vi "Master.vi"() -> ()   [LabVIEW 2025]
doc: "Author: Scott Hannahs <sth@magnet.fsu.edu>\n\nThis software is licensed for use under the “MIT License\"\nCopyright (c) 2025 Scott Hannahs, sth@sth@magnet.sthnet.net\n\nPermission is hereby granted, free of charge, to any person obtaining a copy of this software and associated documentation files (the \"Software\"), to deal in the Software without restriction, including without limitation the rights to use, copy, modify, merge, publish, distribute, sublicense, and/or sell copies of the Software, and to permit persons to whom the Software is furnished to do so, subject to the following conditions: The above copyright notice and this permission notice shall be included in all copies or substantial portions of the Software.\n\nTHE SOFTWARE IS PROVIDED \"AS IS\", WITHOUT WARRANTY OF ANY KIND, EXPRESS OR IMPLIED, INCLUDING BUT NOT LIMITED TO THE WARRANTIES OF MERCHANTABILITY, FITNESS FOR A PARTICULAR PURPOSE AND NONINFRINGEMENT. IN NO EVENT SHALL THE AUTHORS OR COPYRIGHT HOLDERS BE LIABLE FOR ANY CLAIM, DAMAGES OR OTHER LIABILITY, WHETHER IN AN ACTION OF CONTRACT, TORT OR OTHERWISE, ARISING FROM, OUT OF OR IN CONNECTION WITH THE SOFTWARE OR THE USE OR OTHER DEALINGS IN THE SOFTWARE."
uses:
  Globals and TypeDefs/Type Definitions.llb/CCDParameter.ctt
  Globals and TypeDefs/Type Definitions.llb/FileFormatParameter.ctt
  Globals and TypeDefs/Type Definitions.llb/FilePathParameter.ctt
  Globals and TypeDefs/Type Definitions.llb/FileInfoParameter.ctt
  Globals and TypeDefs/Type Definitions.llb/Wavelength Unit.ctt
  Globals and TypeDefs/Type Definitions.llb/McPherson Grating Density.ctl
  Globals and TypeDefs/Type Definitions.llb/OperationMode.ctt
  Globals and TypeDefs/Type Definitions.llb/ListOfDetectors.ctt
  Globals and TypeDefs/Type Definitions.llb/3 way Status.ctl
  LV7/OpticsSS.ctl
  LV7/PlottSS.ctl
  Globals and TypeDefs/gStatus.vi
  Instance          41 14Saved   Master .vi
  Globals and TypeDefs/gDetector.vi
  Globals and TypeDefs/gGeneral.vi
  Sub VIs/File and save/X-Axis Converter.llb/X-Axis Converter.vi
  Globals and TypeDefs/gHField.vi
panel:
  in  "Case Constant\n(See Context Help) 2":bool=TRUE
  in  "Case Constant\n(See Context Help)":bool
  in  "Stop-All":bool
  in  "Prefix_indexed":bool
  out "Path array":path[](array[path])
  out "PDA Temperature":dbl(graph)
  out "#PixelOverflow":u32
  out "Pixel Overflow":bool
  out "Error":errorcluster
  out "Master State":T1=enum."Init"
  in  "EngageTime":bool
  in  "ExpTimeTarget":dbl=12.0
  in  "SaveData?":bool
  in  "Print?":bool
  out "Operation Mode":T2
  in  "SubFolderNamesArray":string[](array[string])
  in  "HTL Array":dbl[][](array[numeric])
  in  "LoadData?":bool
  out "Field":T3 caption="H" items=["N.A.", "OK", "Busy", "Done"]
  out "Tmeperature":T3 caption="T" items=["N.A.", "OK", "Busy", "Done"]
  out "Spectrometer":T3 caption="l" items=["N.A.", "OK", "Busy", "Done"]
  out "Exposure time display":dbl(slide)=0.133 caption="Exposure" scale=0.0..0.2 scale format="%.1f"
  out "Elapsed Time":string
  out "Status Message Board":string="Welcome to NHMFL!\nVisible Optics\nProgram"
  in  "Check Prefix?":bool
  in  "SetDirectory?":bool
  in  "Y Data":dbl[](array[numeric])=[4.359859227115864, 4.389200892828675, 4.418863708420512, 4.448852482615925, 4.479172114380057, 4.509827594937488, 4.540824009842933, 4.572166541105726, 4.6038604693694944, 4.635911176148454, 4.668324146122441, 4.701104969491852, 4.734259344394734, 4.767793079387671, 4.801712095992179, 4.83602243130902, 4.870730240701915, 4.905841800553186, 4.941363511093324, 4.97730189930649, 5.0136636219147634, 5.050455468442887, 5.087684364366512, 5.125357374346244, 5.16348170554992, 5.202064711066347, 5.241113893412698, 5.280636908138933, 5.320641567532123, 5.361135844423454, 5.40212787610175, 5.443625968336108, 5.485638599511655, 5.528174424881744, 5.571242280940019, 5.614851189916724, 5.659010364402478, 5.703729212104152, 5.749017340736845, 5.79488456305601, 5.8413409020348865, 5.888396596191121, 5.936062105068024, 5.984348114875219, 6.033265544293544, 6.082825550450229, 6.133039535069095, 6.1839191508021365, 6.235476307748183, 6.287723180164464, 6.340672213378188, 6.394336130903802, 6.44872794177352, 6.5038609480878895, 6.55974875279337, 6.616405267695311, 6.673844721713221, 6.732081669387259, 6.79113099964405, 6.851007944830221, 6.9117280900235425, 6.9733073826300265, 7.0357621422775445, 7.099109071015688, 7.1633652638319365, 7.228548219495836, 7.294675851741292, 7.36176650079951, 7.429838945294219, 7.498912414511272, 7.569006601056504, 7.640141673914049, 7.7123382919199805, 7.785617617665268, 7.860001331842512, 7.935511648052952, 8.012171328088485, 8.090003697706326, 8.169032662913095, 8.249282726775652, 8.33077900677827, 8.413547252743905, 8.49761386534048, 8.58300591519227, 8.66975116261715, 8.757878078012872, 8.847415862913794, 8.93839447174277, 9.030844634282277, 9.124797878889435, 9.220286556482478, 9.317343865324164, 9.41600387663149, 9.516301561040184, 9.618272815953393, 9.721954493806981, 9.827384431281825, 9.934601479497585, 10.043645535221685, 10.154557573128157, 10.267379679144385, 10.382155084921548, 10.498928203469083, 10.617744665992642, 10.738651359976075, 10.861696468551548, 10.986929511199559, 11.114401385825383, 11.244164412257609, 11.376272377215363, 11.510780580794803, 11.647745884522498, 11.787226761028752, 11.929283345392315, 12.073977488209161, 12.22137281044176, 12.371534760102007, 12.524530670826199, 12.680429822398747, 12.83930350328164, 13.001225075210728, 13.166270039915263, 13.33451610802253, 13.506043270206384, 13.680933870638214, 13.859272682802093, 14.041146987729777, 14.226646654715656, 14.41586422456719, 14.608894995444231, 14.80583711134241, 15.00679165326711, 15.211862733147012, 15.421157590528683, 15.634786692088575, 15.852863833997525, 16.075506247159804, 16.302834705347756, 16.534973636240313, 16.77205123536335, 17.014199582923293, 17.261554763504943, 17.51425698859712, 17.77245072188844, 18.036284807256397, 18.3059125993568, 18.58149209668873, 18.863186076991337, 19.15116223479378, 19.445593320905605, 19.746657283603096, 20.054537411216362, 20.369422475784297, 20.691506877387, 21.02099078870748, 21.35808029931693, 21.702987559097092, 22.0559309201451, 22.417135076413132, 22.786831200239348, 23.165257074828247, 23.552657221611106, 23.949283021300772, 24.35539282730692, 24.771252070023422, 25.197133350337953, 25.63331652051566, 26.080088750418582, 26.537744576792313, 27.006585933108887, 27.486922157200187, 27.979069973614642, 28.48335344733274, 29.000103905129734, 29.52965982050742, 30.072366657732513, 30.628576670076946, 31.198648646914766, 31.78294760382926, 32.38184440935961, 32.99571534146977, 33.624941566211746, 34.26990853044752, 34.931005259824005, 35.60862355250491, 36.3031570584605, 37.01500023335454, 37.74454715533088, 38.49219019221989, 39.25831850591429, 40.04331637991872, 40.847561355318334, 41.67142215974196, 42.51525641324812, 43.37940809451772, 44.26420475032537, 45.169954430957425, 46.09694233418251, 47.04542714051036, 48.015637022906574, 49.00776531492666, 50.02196582239054, 51.05834776541544, 52.11697033983435, 53.19783688989854, 54.30088868779076, 55.42599831987955, 56.57296268504168, 57.74149561674433, 58.931220148080584, 60.1416604476788, 61.37223346434939, 62.622240329675115, 63.890857580390986, 65.17712827640742, 66.4799531056599, 67.79808158341963, 69.1301034712415, 70.47444055896403, 71.82933897185566, 73.19286218368788, 74.56288493456158, 75.93708826921247, 77.31295592634606, 78.68777232151824, 80.05862237420615, 81.42239343285824, 82.77577954893358, 84.11528834098996, 85.43725067181454, 86.73783333448564, 88.0130549062849, 89.25880488223545, 90.4708661424704, 91.64494074005955, 92.77667891917588, 93.86171118887495, 94.89568318741601, 95.87429297840674, 96.79333032630886, 97.64871740856572, 98.43655033863818, 99.15314080272404, 99.79505705677101, 100.35916349333694, 100.84265797303367, 101.24310612502882, 101.55847185679316, 101.78714337508754, 101.92795410705088, 101.98019801980197, 101.94363896561752, 101.81851382289437, 101.60552935527126, 101.30585286653462, 100.92109688110092, 100.4532982230126, 99.90489199503531, 99.27868106899476, 98.57780178535918, 97.80568662187997, 96.96602462681605, 96.06272042200558, 95.09985256623146, 94.08163203227065, 93.01236149485176, 91.89639605523514, 90.73810594515385, 89.54184166257876, 88.31190189802533, 87.05250451647399, 85.76776076963034, 84.461652828644, 83.13801465065819, 81.8005161249856, 80.4526503871352, 79.09772414177037, 77.73885079871027, 76.37894619898024, 75.02072668985214, 73.66670929786417, 72.31921374603169, 70.98036606460397, 69.65210355285129, 68.33618086133153, 67.03417697891065, 65.74750292571056, 64.47740997120414, 63.22499821536264, 61.99122538944135, 60.77691575122682, 59.582768967111335, 58.40936888981143, 57.25719215587677, 56.12661654114332, 55.017929024924804, 53.93133352507879, 52.86695827602707, 51.82486283053664, 50.80504467356964, 49.807445442875476, 48.831956756394504, 47.87842565094678, 46.94665964030745, 46.036431403641515, 45.14748311748012, 44.27953044611727, 43.43226620646358, 42.6053637241895, 41.79847989842212, 41.011257992390064, 40.243330167348105, 39.49431977680977, 38.763843437704175, 38.05151289452863, 37.356936691921696, 36.67972167041139, 36.01947429933415, 35.37580186017517, 34.74831349280977, 34.13662111634363, 33.540340235512275, 32.959090642839186, 32.39249702604861, 31.840189489538492, 31.301803998049735, 30.7769827500592, 30.265374487814174, 29.76663475037882, 29.28042607553899, 28.80641815591104, 28.344287954158954, 27.893719781782664, 27.454405345555568, 27.026043765322786, 26.608341566525006, 26.201012650514798, 25.803778245431467, 25.41636684014538, 25.03851410354023, 24.669962791171823, 24.31046264115136, 23.95977026090333, 23.61764900628636, 23.28386885441087, 22.95820627133951, 22.640444075739502, 22.330371299429107, 22.027783045661604, 21.73248034589445, 21.444270015698585, 21.16296451039404, 20.888381780917932, 20.620345130372943, 20.35868307164673, 20.10322918643533, 19.853821985965663, 19.61030477366188, 19.372525509968213, 19.140336679507016, 18.913595160715975, 18.692162098089153, 18.475902777115053, 18.26468650198858, 18.058386476154528, 17.856879685719345, 17.660046785759945, 17.467771989538537, 17.279942960625498, 17.09645070792191, 16.917189483561163, 16.742056683667286, 16.570952751935298, 16.403781085997196, 16.240447946532107, 16.080862369071976, 15.924936078455998, 15.772583405879114, 15.623721208481035, 15.478268791420303, 15.336147832373733, 15.197282308405232, 15.061598425142755, 14.929024548204785, 14.799491136817574, 14.672930679561734, 14.549277632191464, 14.428468357465825, 14.310441066935024, 14.195135764625045, 14.08249419256267, 13.972459778087526, 13.864977582895126, 13.759994253758327, 13.657457974875705, 13.557318421794335, 13.459526716859063, 13.364035386138228, 13.27079831777925, 13.179770721748449, 13.090909090909092, 13.004171163395661, 12.91951588624077, 12.836903380214224, 12.75629490583483, 12.677652830515154, 12.600940596803213, 12.526122691683634, 12.453164616903683, 12.38203286029049, 12.312694868025606, 12.24511901784625, 12.179274593141457, 12.115131757913815, 12.05266153257834, 11.99183577056985, 11.932627135733041, 11.87500908046845, 11.818955824609674, 11.76444233500797, 11.711444305800104, 11.65993813933795, 11.60990092775727, 11.561310435165108, 11.514145080425847, 11.468383920525726, 11.424006634497912, 11.380993507889265, 11.339325417751663, 11.298983818141277, 11.259950726108972, 11.222208708166901, 11.185740867215678, 11.150530829917827, 11.116562734503766, 11.083821218996304, 11.052291409841342, 11.021958910931758, 10.992809793012693, 10.964830583456795, 10.938008256397914, 10.912330223212965, 10.887784323341283, 10.864358815431716, 10.842042368808027, 10.820824055243078, 10.800693341033405, 10.781640079365355, 10.763654502964759, 10.746727217022421, 10.730849192387653, 10.716011759022894, 10.702206599712252, 10.689425744017434, 10.677661562474725, 10.666906761026693, 10.657154375683012, 10.648397767404552, 10.640630617205472, 10.633846921468175, 10.628040987466086, 10.623207429089685, 10.619341162771164, 10.616437403603506, 10.61449166164985, 10.613499738439238, 10.613457723645045, 10.614361991942566, 10.616209200042398, 10.61899628389644, 10.622720456073516, 10.627379203301786, 10.632970284175236, 10.639491727021781, 10.646941827930538, 10.65531914893617, 10.664622516358094, 10.674851019292753, 10.68600400825716, 10.698081093981964, 10.711082146352725, 10.725007293497864, 10.73985692102218, 10.755631671384794, 10.77233244342051, 10.789960392003877, 10.808516927855083, 10.828003717487244, 10.848422683294594, 10.869776003781105, 10.892066113929618, 10.91529570571105, 10.939467728734005, 10.96458539103486, 10.990652160008423, 11.01767176347996, 11.045648190918651, 11.074585694793534, 11.104488792072516, 11.135362265865236, 11.167211167211168, 11.20004081701363, 11.233856808121402, 11.268665007559191, 11.304471558908258, 11.341282884839375, 11.379105689799312, 11.41794696285327, 11.457813980685149, 11.498714310757618, 11.540655814634878, 11.583646651469962, 11.62769528165972, 11.672810470670129, 11.719001293034513, 11.766277136528466, 11.814647706523917, 11.864123030526423, 11.914713462898968, 11.966429689775758, 12.019282734170648, 12.073283961283387, 12.12844508400873, 12.184778168652574, 12.242295640859474, 12.301010291757152, 12.360935284322133, 12.42208415997257, 12.48447084539341, 12.548109659599271, 12.613015321241827, 12.679202956166797, 12.746688105227863, 12.815486732363786, 12.885615232945288, 12.957090442399794, 13.029929645120367, 13.104150583667508, 13.179771468271484, 13.256810986643078, 13.335288314102453, 13.415223124033782, 13.496635598676047, 13.579546440259186, 13.66397688249509, 13.749948702434974, 13.837484232702424, 13.926606374114439, 14.017338608701486, 14.109705013137976, 14.203730272596845, 14.299439695039455, 14.396859225955392, 14.4960154635654, 14.596935674501095, 14.699647809977643, 14.804180522472912, 14.910563182930376, 15.018825898501593, 15.128999530844538, 15.241115714996932, 15.355206878840859, 15.471306263179047, 15.589447942441705, 15.709666846043369, 15.831998780412336, 15.956480451712276, 16.08314948928004, 16.212044469802226, 16.343204942253628, 16.47667145362424, 16.612485575458262, 16.750689931233456, 16.89132822460762, 17.034445268559747, 17.180087015457268, 17.328300588077308, 17.479134311615432, 17.632637746713556, 17.78886172353971, 17.9478583769566, 18.109681182812103, 18.274384995391078, 18.442026086065923, 18.612662183184362, 18.786352513237837, 18.963157843349737, 19.143140525129375, 19.326364539935806, 19.51289554559672, 19.70280092463277, 19.896149834033558, 20.09301325663871, 20.29346405417522, 20.49757702200397, 20.705428945633606, 20.917098659055448, 21.13266710496104, 21.35221739690145, 21.57583488344913, 21.803607214428858, 22.03562440927946, 22.27197892761611, 22.51276574206055, 22.758082413407966, 23.008029168205347, 23.262708978810554, 23.522227646009927, 23.786693884269244, 24.056219409693583, 24.3309190307785, 24.610910742027375, 24.896315820519412, 25.187258925508026, 25.483868201129862, 25.786275382310958, 26.09461590394749, 26.409029013447665, 26.729657886715053, 27.05664974765271, 27.39015599127249, 27.73033231048255, 28.077338826633632, 28.431340223896083, 28.79250588753546, 29.161010046158022, 29.537031917981217, 29.920755861189793, 30.31237152842447, 30.71207402544193, 31.120064073983663, 31.536548178868856, 31.961738799326668, 32.395854524562374, 32.83912025353589, 33.291767378922756, 33.75403397519474, 34.22616499074848, 34.70841244397801, 35.20103562315853, 35.70430128998762, 36.21848388658109, 36.743865745697, 37.2807373039094, 37.82939731740552, 38.39015308003834, 38.96332064319138, 39.54922503696516, 40.14820049211286, 40.76059066207344, 41.386748844375965, 42.0270382005743, 42.681831973785435, 43.35151370277646, 44.03647743141852, 44.73712791219888, 45.453880802309456, 46.18716285068311, 46.937412074152704, 47.705077920707076, 48.49062141761412, 49.29451530191956, 50.11724413059322, 50.95930436729756, 51.821204442444625, 52.70346478289072, 53.60661780723075, 54.53120788228832, 55.47779123595873, 56.44693582110416, 57.43922112472759, 58.45523791609419, 59.495587926931485, 60.56088345621398, 61.651746891388925, 62.76881013723119, 63.91271394274945, 65.08410711582407, 66.28364561441893, 67.51199150234996, 68.76981175672066, 70.05777691316518, 71.37655953411455, 72.72683248428955, 74.1092669966185, 75.52453051079203, 76.97328426561938, 78.45618062540582, 79.97386011959668, 81.52694817404465, 83.11605151148629, 84.7417541980828, 86.4046133123965, 88.10515421280739, 89.84386537927608, 91.62119280559367, 93.43753391876069, 95.29323100317171, 97.1885641087292, 99.12374342407416, 101.0989010989011, 103.11408250278154, 105.16923691237619, 107.26420762426427, 109.39872149710654, 111.5723779346085, 113.78463732972462, 116.03480900108816, 118.32203866462099, 120.64529549690151, 123.0033588622068, 125.39480479205825, 127.81799232482636, 130.27104983316252, 132.75186148874656, 135.25805403686783, 137.78698407721993, 140.33572607186628, 142.90106132583995, 145.47946820982128, 148.0671139170434, 150.65984806694533, 153.2531984854103, 155.84236950429036, 158.4222431302903, 160.98738343390016, 163.53204450143193, 166.05018227635358, 168.53547058854588, 170.9813216309795, 173.38091109184288, 175.72720808570307, 178.01300995009646, 180.23098188419874, 182.37370130512846, 184.43370668665264, 186.40355052675318, 188.27585596792636, 190.0433764705767, 191.6990578197283, 193.23610163304818, 194.64802943849332, 195.92874630773915, 197.0726029712699, 198.0744553067754, 198.92972008756837, 199.6344259043045, 200.1852582325435, 200.5795977101961, 200.81555081101075, 200.89197224975223, 200.80847862709987, 200.5654530119324, 200.16404035900476, 199.60613386401218, 198.89435255837313, 198.0320106357045, 197.02307917433632, 195.87214106971265, 194.58434011263304, 193.16532524079693, 191.6211910503684, 189.95841568084745, 188.18379718160273, 186.30438943418605, 184.32743864427007, 182.2603213348983, 180.11048467305204, 177.885389849312, 175.5924591102524, 173.23902691969622, 170.83229560237197, 168.37929570520407, 165.88685120068226, 163.3615495556608, 160.8097165991903, 158.23739604580024, 155.6503334662017, 153.0539644459122, 150.45340663317825, 147.85345535000155, 145.25858242321343, 142.67293788490863, 140.10035419216482, 137.5443526233475, 135.0081515211617, 132.4946760699316, 130.0065693149577, 127.54620415450763, 125.11569605897792, 122.71691629626862, 120.35150546699153, 118.0208871769936, 115.72628169770708, 113.46871948655841, 111.24905445988026, 109.06797692949733, 106.92602613107003, 104.82360228761749, 102.76097816526601, 100.7383100902379, 98.7556484066402, 96.81294736358653, 94.91007442793571, 93.04681902541851, 91.22290071827247, 89.43797683196064, 87.69164954700636, 85.98347247475698, 84.31295673795266, 82.67957657842356, 81.08277451527354, 79.52196607740966, 77.99654413451097, 76.50588285043271, 75.04934128267388, 73.62626665105351, 72.23599729800955, 70.87786536216365, 69.55119918590644, 68.25532547678353, 66.989571241518, 65.75326551045683, 64.54574086924336, 63.36633481351214, 62.21439094139057, 61.089259997666595, 59.99030078251254, 58.91688093678181, 57.8683776150366, 56.84417805662603, 55.84368006439242, 54.86629239981791, 53.911435102754524, 52.97853974323218, 52.06704961221306, 51.17641985762386, 50.306117571439195, 49.45562183311679, 48.624423714227504, 47.812026248683935, 47.01794437260552, 46.24170483747118, 45.48284609989282, 44.74091819103539, 44.01548256841131, 43.306111952540896, 42.61239015070839, 41.933911869839505, 41.270282520325516, 40.62111801242236, 39.986044546706715, 39.364698399897456, 38.75672570722455, 38.16178224240005, 37.579533196118035, 37.0096529539243, 36.451824874181916, 35.90574106678451, 35.37110217318958, 34.847617148262465, 34.335003044374055, 33.83298479812016, 33.341295019989, 32.85967378725514, 32.38786844032609, 31.92563338274469, 31.472729885000874, 31.028925892285255, 30.59399583628902, 30.167720451121262, 29.749886593406902, 29.340287066594833, 28.938720449497826, 28.54499092906973, 28.15890813740441, 27.780286992941413, 27.408947545840558, 27.044714827486775, 26.687418704078205, 26.3368937342368, 25.992979030586355, 25.65551812522657, 25.324358839035185, 24.999353154726343, 24.680357093584345, 24.367230595799825, 24.059837404323954, 23.758044952161082, 23.461724253019675, 23.170749795234723, 22.884999438884304, 22.60435431601352, 22.328698733885684, 22.05792008118085, 21.791908737057103, 21.53055798299983, 21.27376391737627, 21.021425372619895, 20.773443834969687, 20.529723366686287, 20.290170530675923, 20.054694317446987, 19.82320607433054, 19.595619436897397, 19.371850262501688, 19.151816565889344, 18.93543845680471, 18.722638079534455, 18.513339554329608, 18.30746892064386, 18.104954082134622, 17.90572475336819, 17.709712408176312, 17.51685022961275, 17.327073061456208, 17.140317361213445, 16.956521154571956, 16.77562399125692, 16.597566902248243, 16.42229235831149, 16.249744229803607, 16.07986774770962, 15.912609465871899, 15.747917224374362, 15.585740114042, 15.4260284420226, 15.26873369841338, 15.113808523899822, 14.961206678374843, 14.810883010504563, 14.662793428212746, 14.51689487005212, 14.373145277435007, 14.231503567696258, 14.091929607959841, 13.954384189785666, 13.818829004569535, 13.685226619673003, 13.553540455260446, 13.423734761818881, 13.295774598341003, 13.169625811148363, 13.045255013335167, 12.922629564813562, 12.801717552939623, 12.682487773703725, 12.56490971346569, 12.448953531218253, 12.334590041362802, 12.221790696979657, 12.110527573579299, 12.000773353317886, 11.892501309663155, 11.785685292497277, 11.68029971364149, 11.5763195327913, 11.4737202438479, 11.372477861634222, 11.272568908984288, 11.173970404192929, 11.076659848816483, 10.980615215812294, 10.885814938007247, 10.792237896885748, 10.699863411686152, 10.608671228797805, 10.518641511448305, 10.429754829672692, 10.341992150556594, 10.255334828743806, 10.169764597201846, 10.085263558236575, 10.001814174748855, 9.919399261726573, 9.838001977963811, 9.757605818001839, 9.678194604284215, 9.599752479520156, 9.522263899250422, 9.445713624608777, 9.370086715274489, 9.295368522609328, 9.22154468297399, 9.148601111219307, 9.076523994345967, 9.00529978532927, 8.934915197103027, 8.865357196698499, 8.79661299953429, 8.728670063851933, 8.661516085294144, 8.595138991620736, 8.529526937558694, 8.464668299782959, 8.400551672023308, 8.337165860294927, 8.274499878248228, 8.212542942635004, 8.151284468887964, 8.090714066809685, 8.030821536368922, 7.971596863600483, 7.913030216606138, 7.855111941654126, 7.797832559373704, 7.741182761043143, 7.685153404967791, 7.629735512946082, 7.574920266821415, 7.520699005116799, 7.467063219750945, 7.4140045528328695, 7.361514793533171, 7.309585875030267, 7.258209871528803, 7.207378995349226, 7.157085594085887, 7.107322147832155, 7.058081266471045, 7.009355687028948, 6.961138271091613, 6.913422002280089, 6.866199983785316] format="%.4f"
  in  "File Info":T4={"FilePath"=path "/Volumes/DATA/Labview Items", "Field (T)"=55.0, "Temperature (K)"=77.0, "X-Axis"=enum."nm", "Center nm"=55.0, "Current Grating Density"=enum."600", "CCD Parameters"={"Exposure Time (s)"=0.2, "Offset"=0.0, "BkgrdCrct"=FALSE, "Shutter"=FALSE, "Mode"=enum."Regular", "Repetition"=4, "dt or s"=0.0}, "Operation Mode"=enum."NML Data Acquisition", "Exp Index"=0, "Index_repetition"=0, "Index"=0, "Current Detector"=enum."CCD-1024x256"} {"CCD Parameters"."dt or s" format="%#.6f"; "CCD Parameters"."Repetition" min=1; "CCD Parameters"."Offset" format="%#.2f"; "CCD Parameters"."Exposure Time (s)" min=0.02 max=6000.0 format="%#.2f"; "Center nm" format="%.2f"; "Temperature (K)" format="%.2f"; "Field (T)" format="%.2f"}
  out "Most recently saved file":path=path "erererere"
  in  "FilePath_C":T9={"Filename Prefix"="MyData", "Extension"=enum."±Field", "Suffix"="", "Current Path"=path "/Volumes/Cell06DataMac/Users/Shared/Data"}
  in  "User Comments":string="This data's for you!\nThis is where the experimenter can write random, rambling comments that will never be looked at but will be stored (if you choose so) for all eternity with the data file header."
  in  "Main Tab":T10(tab)
  in  "ShowRange":bool
  in  "CCD Parameters":T7={"Exposure Time (s)"=0.2, "Offset"=580.0, "BkgrdCrct"=FALSE, "Shutter"=TRUE, "Mode"=enum."Regular", "Repetition"=1, "dt or s"=0.0} {"dt or s" format="%#.6f"; "Repetition" min=1; "Offset" format="%#.2f"; "Exposure Time (s)" min=0.02 max=6000.0 format="%#.2f"}
  in  "CCD Control Tab":T11(tab)
  in  "AutoSaveData":bool
  in  "BkgrdShot":bool
  in  "nextShot":bool caption="Shot"
  in  "CancelSeq?":bool
  in  "Park Seq":bool caption="Park after exp?"
  in  "PauseSeq?":bool
  in  "startSeq?":bool
  in  "RampSelect":bool[](array[boolean])=[TRUE, TRUE, FALSE, FALSE, FALSE, FALSE]
  in  "HRamp Paras":dbl[][](array[numeric])=[[0.0, 30.0, 1.0, 20.0], [30.0, 0.0, -1.0, 20.0], [0.0, -30.0, -1.0, 20.0], [-30.0, 0.0, 1.0, 20.0], [0.0, 30.0, 0.5, 20.0], [30.0, 0.0, -0.5, 20.0]] step=1.0 format="%.2f"
  in  "CancelCustSeq?":bool
  in  "Park Cust Seq":bool caption="Park after exp?"
  in  "Cust Seq Para Setup":bool
  in  "PauseCustSeq?":bool
  in  "startCustSeq?":bool
  in  "Init PDA":bool
  in  "Init CCD":bool
  out "InGaAs OK?":bool
  out "CCD OK?":bool
  in  "Select Detector":enum8{"CCD-1024x256", "InGaAs PDA-1024x1"}(ring)
  in  "CCD LineSet?":bool caption="ldb,1,16,u,0,225,25,b,1,15;sdu,0,1024,1024;cl0;omrm;sron"
  in  "Calibration":bool
  in  "Main Setup Tab":enum32{"General Info", "Expert Setup"}(tab)
  in  "File Format":T12={"File Format"=enum."Macintosh (EOL: CR)", "Delimiter"=enum."TAB", "SaveComments?"=enum."Saved in the Header Area"}
  in  "Data Buffer Size":i16=100 min=10 max=500
  in  "BusScan?":bool
  in  "Graph Tab":T13(tab)
  out "File Info Buffer Out":T4[](array[typedef]) {"CCD Parameters"."dt or s" format="%#.6f"; "CCD Parameters"."Repetition" min=1; "CCD Parameters"."Offset" format="%#.2f"; "CCD Parameters"."Exposure Time (s)" min=0.02 max=6000.0 format="%#.2f"; "Center nm" format="%.2f"; "Temperature (K)" format="%.2f"; "Field (T)" format="%.2f"}
  out "Cursor delta x & y":dbl[](array[numeric])
  in  "Fixed":bool
  out "Pin":bool[](array[boolean])=[FALSE, FALSE, FALSE, FALSE, FALSE, FALSE, FALSE, FALSE, FALSE, TRUE]
  in  "Column Headings":string[](array[string])=["Current", "Previous", "older", "Ref#1", "Ref#2", "Ref#3", "Ref#4", "Ref#5", "Ref#6", "Ref#7"]
  in  "Trace":bool[](array[boolean])=[FALSE, FALSE, FALSE, FALSE, FALSE, FALSE, FALSE, FALSE, FALSE, FALSE]
  in  "X-Axis Unit":u16(ring)=1 items=["Point #", "nanometer (nm)", "electron volt (eV)", "Milli eV (meV)", "Wavenumber (cm-1)"]
  out "Main Data Plot":cluster{dbl[], dbl[]}[](graph)
  in  "FindBPeaks":bool
  in  "FindAPeaks":bool
  out "A peaks: X":dbl[](array[numeric]) format="%#_8g"
  out "A peaks: Y":dbl[](array[numeric]) format="%.3e"
  out "B peaks: X":dbl[](array[numeric]) format="%#_8g"
  out "B peaks: Y":dbl[](array[numeric]) format="%.3e"
  in  "APeakIndex":u16(ring)=4 items=[" 1:  693.402 nm", " 2:  694.827 nm"]
  in  "BPeakIndex":u16(ring)=4 items=[" 1:  693.418 nm", " 2:  694.865 nm"]
  out "DX":dbl caption="kb" format="%.2f"
  in  "Pressure Unit?":bool
  out "Analyis Data Plot":cluster{dbl[], dbl[]}[](graph)
  out "Waveform Graph":dbl[](graph)
  out "Op-Mode":u8(ring) items=["none", " + ", " - ", " * ", " / ", "Integral", "Differential", "FFT"]
  in  "Print IntGraph":bool
  in  "Operation":bool
  in  "Ref Load":bool
  in  "Batch Load":bool
  out "Data IntGraph":dbl[][](graph)
  out "Intensity Graph":i32[][](graph)
  # "l"
  # "Filename Prefix"
  # "Extension"
  # "Suffix"
  # "Select   StartField (T)   EndField (T)   FieldStep (T)"
  # "To be constructed"
  # "To be constructed"
  # "Peak#   Position   Intensity"
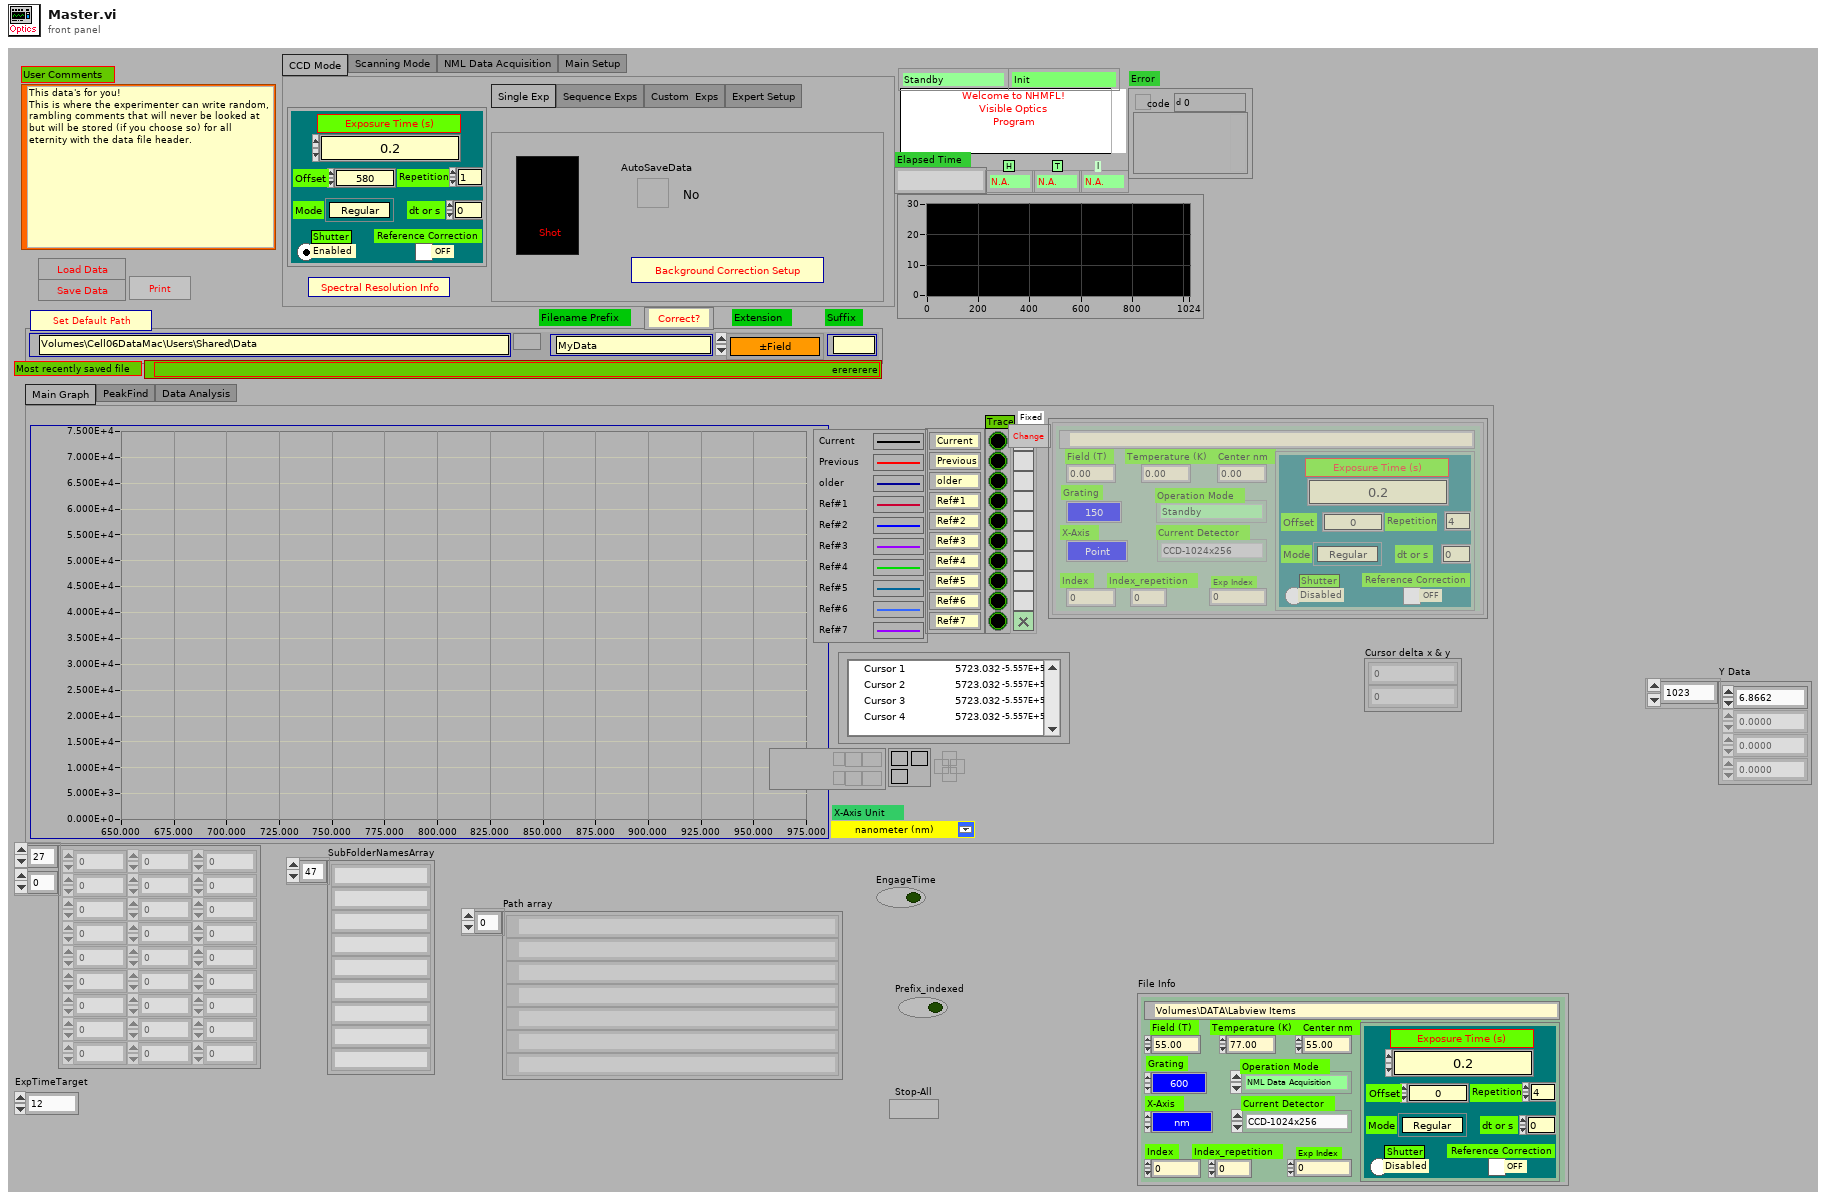
[diagram p1: front panel]
types:
  T1 = typedef "OpticsSS.ctl" = enum16{"_Quit_", "Init", "Ready", "HTL", "CCD_shot", "QueueData", "Error Handler", "HTL Error", "CCD Error", "CCDSetup", "Calibration", "BG_Setup", "HTL Paras Setup"}
  T2 = typedef "OperationMode.ctt" = enum16{"Standby", "CCD Single Shot", "CCD Sequence Shots", "CCD Custom Shots", "CCD Reference Shot", "Step Scanning ", "Time Scanning", "NML Data Acquisition"}
  T3 = typedef "3 way Status.ctl" = u8
  T4 = typedef "FileInfoParameter.ctt" = cluster{"FilePath":path, "Field (T)":dbl, "Temperature (K)":dbl, "X-Axis":T5, "Center nm":dbl, "Current Grating Density":T6, "CCD Parameters":T7, "Operation Mode":T2, "Exp Index":u32, "Index_repetition":u16, "Index":u16, "Current Detector":T8}
  T5 = typedef "Wavelength Unit.ctt" = enum8{"Point", "nm", "eV", "meV", "cm_1"}
  T6 = typedef "McPherson Grating Density.ctl" = enum8{"150", "300", "600", "1200", "1800"}
  T7 = typedef "CCDParameter.ctt" = cluster{"Exposure Time (s)":dbl, "Offset":dbl, "BkgrdCrct":bool, "Shutter":bool, "Mode":enum8{"Regular", "OverExp Cor", "SpikeRemove", "ForCalibration"}, "Repetition":u16, "dt or s":dbl}
  T8 = typedef "ListOfDetectors.ctt" = enum8{"CCD-1024x256", "InGaAs PDA-1024x1", "CCD-1340x400", "Ge Single Channel", "Si Single Channel", "PMT Single Channel"}
  T9 = typedef "FilePathParameter.ctt" = cluster{"Filename Prefix":string, "Extension":enum16{"none", "\".001\",\".002\", ...", "001 (No dot)", "±Field", "pField nField", "Temperature", "Wavelength", "T(K)±H(T)", "(nm)T(K)±H(T)", "User Defined"}, "Suffix":string, "Current Path":path}
  T10 = enum32{"CCD Mode", "Scanning Mode", "NML Data Acquisition", "Main Setup"}
  T11 = enum32{"Single Exp", "Sequence Exps", "Custom  Exps", "Expert Setup"}
  T12 = typedef "FileFormatParameter.ctt" = cluster{"File Format":enum16{"Macintosh (EOL: CR)", "Unix (EOL: LF)", "DOS/Windows (EOL: CR+LF)"}, "Delimiter":enum16{"TAB", "COMMA", "SPACE"}, "SaveComments?":enum16{"Bare data only", "Saved in the Header Area", "Saved as a Parameter File"}}
  T13 = enum32{"Main Graph", "PeakFind", "Data Analysis"}
  T14 = enum16{"--Quit--", "Init GPIB", "Poll GPIB", "Wait for SRQ", "Clear CCD Parameters", "New CCD Parameters", "Check CCD Command Error"}
  T15 = cluster{"Exposure (ms)":u32, "Interval (ms)":u32, "Flush Count":i32, "Trigger":u16}
  T16 = enum16{"End", "Init", "Reset", "SetAcqParameter", "SetArea", "Start Acquisition", "Busy Status Poll", "Read", "Stop"}
  T17 = enum16{"Pass", "Write", "Read", "ReadPlotBlock", "Initialize", "InitFromBufferInput", "Resize Buffer"}
  T18 = enum32{"existing file", "new file", "new or existing file", "existing dir", "new dir", "new or existing dir", "existing file (use LLBs)", "new file (use LLBs)", "new or existing file (use LLBs)", "new or existing file or directory (use LLBs)"}
  T19 = enum16{"none", "\".001\",\".002\", ...", "001 (No dot)", "±Field", "pField nField", "Temperature", "Wavelength", "T(K)±H(T)", "(nm)T(K)±H(T)", "User Defined"}
  T20 = enum16{"none", " + ", " - ", " * ", " / ", "Integral", "Differential", "FFT"}
  T21 = typedef "PlottSS.ctl" = enum16{"_Quit_", "Init", "load", "Pin-Mix", "Trace-Show/Hide", "Unit-Change", "Display/Print", "Column Heading"}
  T22 = enum16{"The Reference CCD Shot", "The Reference File", "The Constant", "Current Reference"}
  T23 = enum16{"Auto Data Saving", "Manual Data Saving", "Auto Sequence Saving", "Sequence Saving from Data Buffer"}
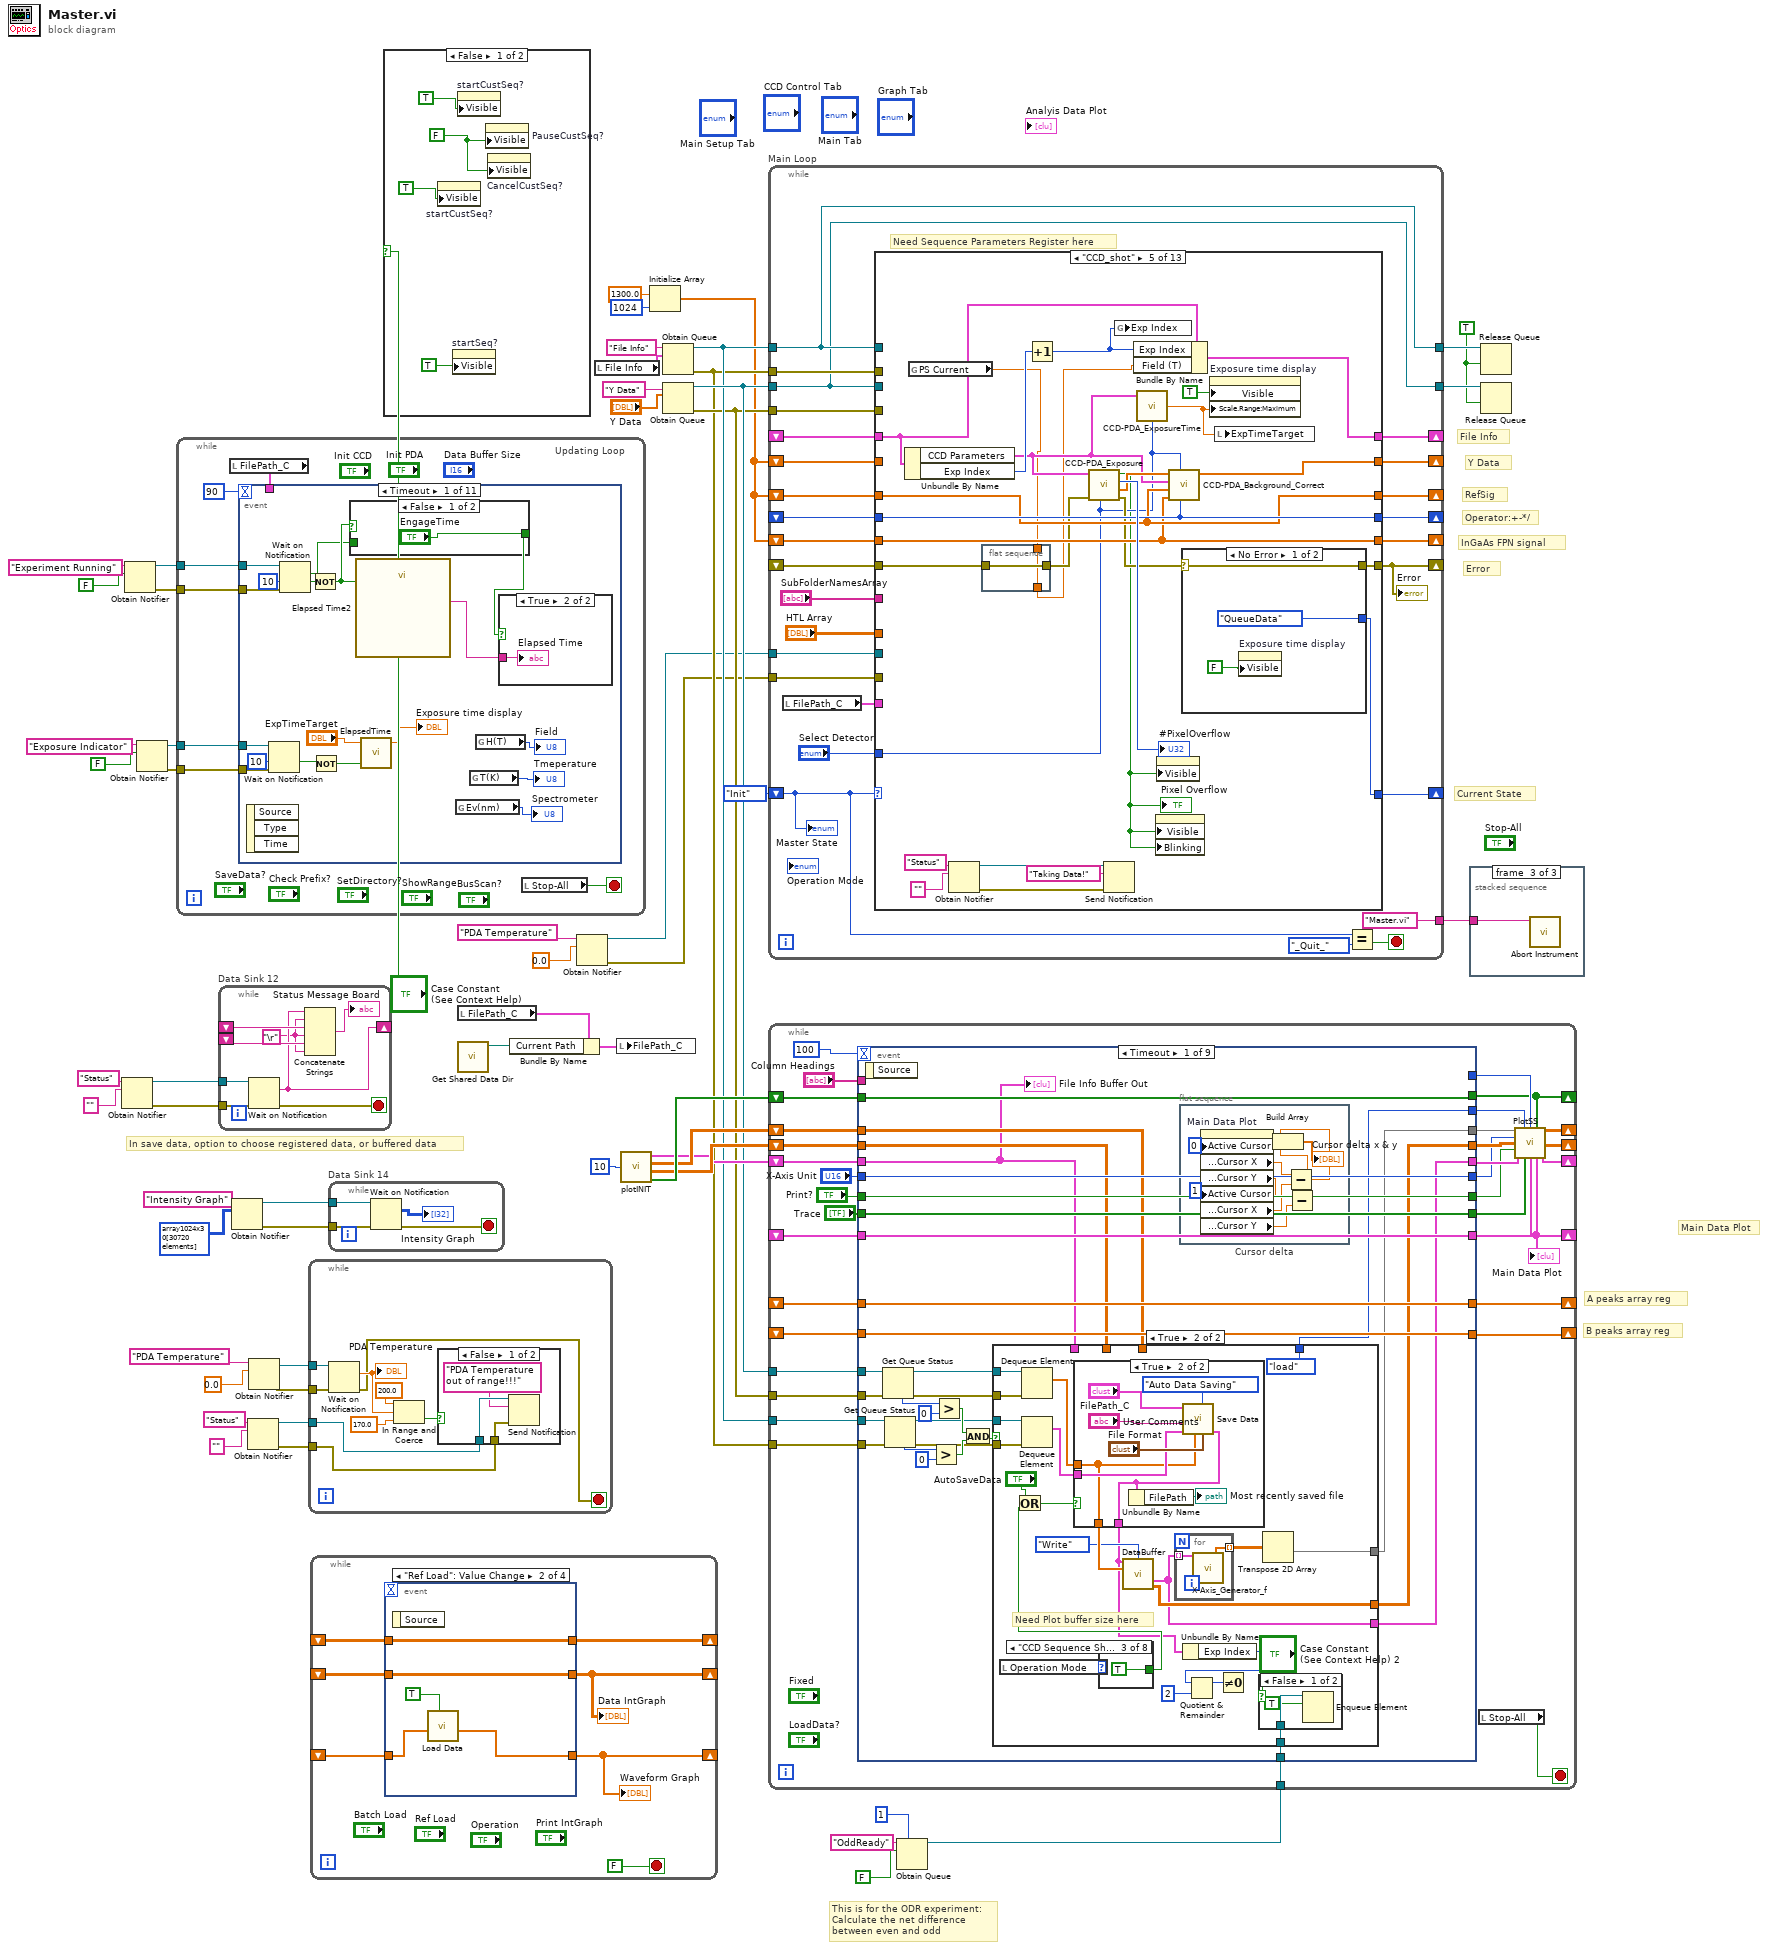
[diagram p0: block diagram]
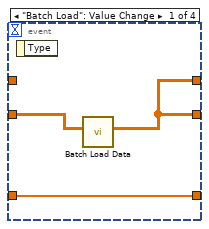
[diagram p2: hidden frame]
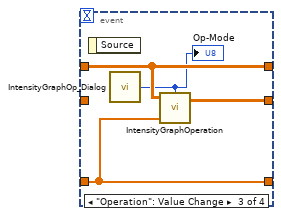
[diagram p3: hidden frame]
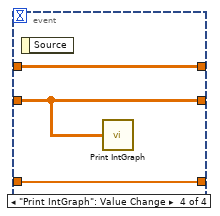
[diagram p4: hidden frame]
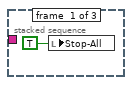
[diagram p5: hidden frame]
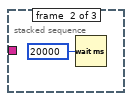
[diagram p6: hidden frame]
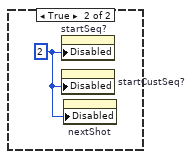
[diagram p8: hidden frame]
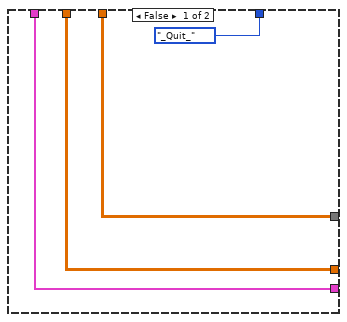
[diagram p9: hidden frame]
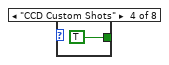
[diagram p13: hidden frame]
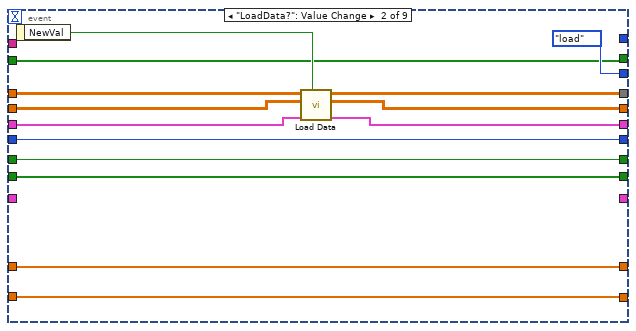
[diagram p19: hidden frame]
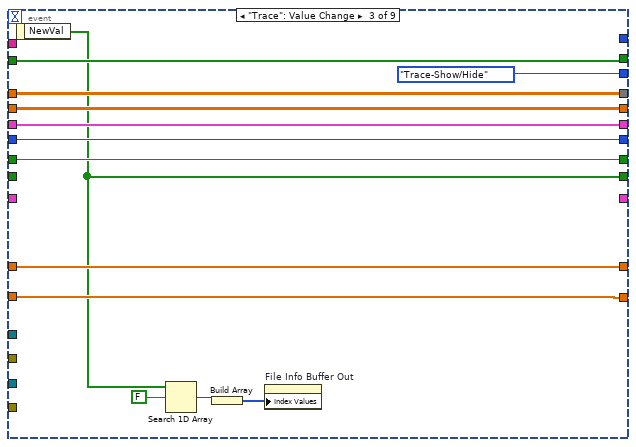
[diagram p20: hidden frame]
diagram:
  w50 = TRUE ("force destroy? (F)")
  # "This is for the ODR experiment:\nCalculate the net difference \nbetween even and odd"
  # "Current State"
  # "Error"
  # "InGaAs FPN signal"
  # "Operator:+-*/"
  # "RefSig"
  # "Y Data"
  # "File Info"
  # "In save data, option to choose registered data, or buffered data"
  # "B peaks array reg"
  # "A peaks array reg"
  # "Main Data Plot"
  n1 = Obtain Notifier(name (unnamed)="Status", notification data type="" ("Status")) -> (notifier out=w31:refnum<notifier>, error out=w30:errorcluster)  [unwired: 2 in, 1 out]
  n2 = Obtain Notifier(name (unnamed)="Experiment Running", notification data type=FALSE ("SaveData?")) -> (notifier out=w34:refnum<notifier>, error out=w33:errorcluster)  [unwired: 2 in, 1 out]
  n3 = Obtain Notifier(name (unnamed)="Exposure Indicator", notification data type=FALSE ("SaveData?")) -> (notifier out=w38:refnum<notifier>, error out=w37:errorcluster)  [unwired: 2 in, 1 out]
  n4 = while "Updating Loop" {
    tunnel: w38 -> [w62]
    tunnel: w37 -> [w61]
    tunnel: w34 -> [w60]
    tunnel: w33 -> [w59]
    stop <- w58 stop-if-true
    n5 = local read "FilePath_C"() -> (w64:T9)
    n6 = event shown="[0] Timeout" {
      selector: _ -> [_ _ _ _ _ _ _ _ _ _ _]
      dyn-events: _ -> [_ _ _ _ _ _ _ _ _ _ _]
      timeout: 90 -> [_ _ _ _ _ _ _ _ _ _ _]
      tunnel: w64 -> [_ _ _ w98 w104 _ w121 _ _ _ _]
      tunnel: w62 -> [w82 _ _ _ _ _ _ _ _ _ _]
      tunnel: w61 -> [w81 _ _ _ _ _ _ _ _ _ _]
      tunnel: w60 -> [w77 _ _ _ _ _ _ _ _ _ _]
      tunnel: w59 -> [w76 _ _ _ _ _ _ _ _ _ _]
      event Timeout {
        n7 = event-data() -> ()  [unwired: 1 in, 3 out]
        n8 = Wait on Notification(notifier=w82, timeout in ms (-1)=10, error in (no error)=w81) -> (timed out?=w79:bool)  [unwired: 1 in, 3 out]
        n9 = Wait on Notification(notifier=w77, timeout in ms (-1)=10, error in (no error)=w76) -> (notification=w73:bool, timed out?=w75:bool)  [unwired: 1 in, 2 out]
        n10 = Not(x=w75) -> (.not. x?=w74:bool)
        n11 = Not(x=w79) -> (.not. x?=w70:bool)
        n12 = case shown="False" w74 {
          tunnel: w73 -> [_ w87]
          tunnel: ["EngageTime" w85] -> w72
          frame False {
          }
          frame True {
            n13 = Select(t=TRUE ("SaveData?"), s=w87, f=FALSE ("SaveData?")) -> (s? t:f=w85:bool)
            n14 = local write "EngageTime"(w85) -> ()
          }
        }
        n15 = call "Elapsed Time2"("Reset"=w74) -> ("Elapsed Time Text"=w68:string)  [unwired: 11 in, 7 out]
        n16 = call "ElapsedTime.vi"("Reset"=w70, "Target time(s)"="ExpTimeTarget") -> ("Elapsed Time"=→"Exposure time display":dbl)  [unwired: 2 in, 1 out]
        n17 = global read "gStatus.vi" "Ev(nm)"() -> (→"Spectrometer":T3)
        n18 = global read "gStatus.vi" "T(K)"() -> (→"Tmeperature":T3)
        n19 = global read "gStatus.vi" "H(T)"() -> (→"Field":T3)
        n20 = case shown="True" w72 {
          tunnel: w68 -> [_ w83]
          frame False {
          }
          frame True {
            "Elapsed Time" <- w83
          }
        }
      }
      event Mouse Down {
        n21 = event-data() -> ()  [unwired: 1 in, 1 out]
        n22 = Obtain Notifier(name (unnamed)="Wakeup", notification data type=TRUE) -> (notifier out=w91:refnum<notifier>, error out=w90:errorcluster)  [unwired: 2 in, 1 out]
        n23 = Send Notification(notification=TRUE, notifier=w91, error in (no error)=w90) -> ()  [unwired: 2 out]
      }
      event "Select Detector": Value Change {
        n24 = event-data() -> ()  [unwired: 1 in, 1 out]
        n25 = local read "Select Detector"() -> (w94:enum8{"CCD-1024x256", "InGaAs PDA-1024x1"})
        n26 = local read "File Info"() -> (w96:T4)
        n27 = global write "gDetector.vi" "Current Detector"(w94) -> ()
        n28 = Bundle By Name(cluster=w96, "CCD Parameters"="CCD Parameters", "Current Detector"=w94) -> (w97:T4)
        n29 = local write "File Info"(w97) -> ()
      }
      event "SetDirectory?": Value Change {
        (unwired) T18."new or existing dir" ("select mode (2)")
        n30 = event-data() -> ()  [unwired: 1 in, 1 out]
        n31 = Unbundle By Name(w98) -> ("Current Path"=w103:path)
        n32 = File Dialog(11:w103) -> (1:w101:bool, 3:w102:path)  [unwired: 6 in, 2 out]
        n33 = Select(t=w103, s=w101, f=w102) -> (s? t:f=w100:path)
        n34 = Bundle By Name(cluster=w98, "Current Path"=w100) -> (w99:T9)
        n35 = local write "FilePath_C"(w99) -> ()
      }
      event "Check Prefix?": Value Change {
        n36 = event-data() -> ()  [unwired: 1 in, 1 out]
        n37 = Unbundle By Name(w104) -> ("Filename Prefix"=w107:string, "Extension"=w105:T19)
        n38 = Equal To 0?(x=w105) -> (x = 0?=w106:bool)
        n39 = case shown="True" w106 {
          tunnel: w107 -> [w111 w114]
          tunnel: [w110 w113] -> w108
          frame False {
            n40 = call "Trim_Filename.vi"("Input string"=w111, "length"=21) -> ("output string"=w110:string)
          }
          frame True {
            n41 = call "Trim_Filename_DOS.vi"("Input string"=w114, "length"=7) -> ("output string"=w113:string)
          }
        }
        n42 = Bundle By Name(cluster=w104, "Filename Prefix"=w108) -> (w109:T9)
        n43 = local write "FilePath_C"(w109) -> ()
      }
      event "ShowRange": Value Change {
        n44 = event-data() -> ()  [unwired: 1 in, 6 out]
        n45 = call "ShowRange.vi"("File Info"="File Info") -> ()  [unwired: 6 in]
      }
      event "SaveData?": Value Change {
        n46 = event-data() -> ()  [unwired: 1 in, 3 out]
        n47 = local read "User Comments"() -> (w119:string)
        n48 = local read "File Format"() -> (w120:T12)
        n49 = call "Save DataBuffer.vi"("File Parameter"=w121, "User Comments"=w119, "FileFormat"=w120) -> ("File Info output"=w118:T4)  [unwired: 12 in]
        n50 = Unbundle By Name(w118) -> ("FilePath"=w117:path)
        n51 = local write "Most recently saved file"(w117) -> ()
      }
      event "BusScan?": Value Change {
        n52 = event-data() -> ()  [unwired: 1 in, 1 out]
        n53 = call "GPIB Bus Scan (for CCD).vi"() -> ()  [unwired: 1 in, 1 out]
      }
      event "Init CCD": Value Change {
        n54 = event-data() -> ()  [unwired: 1 in, 1 out]
        n55 = call "CCD_GPIB_Clear.vi"() -> ("error out"=w129:errorcluster)  [unwired: 5 in]
        n56 = Obtain Notifier(name (unnamed)="Status", notification data type="" ("Status")) -> (notifier out=w127:refnum<notifier>, error out=w128:errorcluster)  [unwired: 2 in, 1 out]
        n57 = call "CCD_Initialization.vi"("error in"=w129, "Starting Action"=T14."Init GPIB") -> ("error out"=w124:errorcluster)  [unwired: 3 in, 4 out]
        n58 = case shown="Error" w124 {
          tunnel: w127 -> [w134 w138]
          tunnel: w128 -> [w133 w137]
          tunnel: [u8 0 ("Disabled") u8 0 ("Disabled")] -> w122
          frame No Error {
            w132 = u8 0 ("Disabled")
            n59 = property on="nextShot" class="Bool"("Disabled"=w132) -> ()  [unwired: 2 in, 2 out]
            n60 = property on="startSeq?" class="Bool"("Disabled"=w132) -> ()  [unwired: 2 in, 2 out]
            n61 = property on="startCustSeq?" class="Bool"("Disabled"=w132) -> ()  [unwired: 2 in, 2 out]
            n62 = Send Notification(notification="Re-Initiate CCD Successful", notifier=w134, error in (no error)=w133) -> ()  [unwired: 2 out]
          }
          frame Error {
            n63 = Send Notification(notification="Oh! No. The CCD Does not work!\nCall Xing Wei @ 4-1060 (O), or 668-0504 (H), or 591-6292 (C)!", notifier=w138, error in (no error)=w137) -> ()  [unwired: 2 out]
          }
        }
        n64 = property on="Init CCD" class="Bool"("Disabled"=u8 2) -> ()  [unwired: 2 in, 2 out]
        n65 = property on="Init CCD" class="Bool"("Disabled"=w122) -> ()  [unwired: 2 in, 2 out]
      }
      event "Init PDA": Value Change {
        n66 = event-data() -> ()  [unwired: 1 in, 1 out]
        n67 = Obtain Notifier(name (unnamed)="Status", notification data type="" ("Status")) -> (notifier out=w144:refnum<notifier>, error out=w143:errorcluster)  [unwired: 2 in, 1 out]
        n68 = call "PDA_RegMode_Acquisition.vi"("StartIng Mode"=T16."Init", "Number of Cycles"=u32 1, "Acquisition Parameters"=T15 {"Exposure (ms)"=100, "Interval (ms)"=10, "Flush Count"=1, "Trigger"=0}) -> ("error out"=w142:errorcluster)  [unwired: 2 in, 3 out]
        n69 = case shown="Error" w142 {
          tunnel: w144 -> [w153 w157]
          tunnel: w143 -> [w152 w156]
          tunnel: [u8 0 ("Disabled") u8 0 ("Disabled")] -> w140
          frame No Error {
            w151 = u8 0 ("Disabled")
            n70 = property on="nextShot" class="Bool"("Disabled"=w151) -> ()  [unwired: 2 in, 2 out]
            n71 = property on="startSeq?" class="Bool"("Disabled"=w151) -> ()  [unwired: 2 in, 2 out]
            n72 = property on="startCustSeq?" class="Bool"("Disabled"=w151) -> ()  [unwired: 2 in, 2 out]
            n73 = Send Notification(notification="Re-Initiate PDA Successful", notifier=w153, error in (no error)=w152) -> ()  [unwired: 2 out]
          }
          frame Error {
            n74 = Send Notification(notification="Oh! No. The InGaAs PDA does not work!\nCall Xing Wei @ 4-1060 (O), or 668-0504 (H), or 591-6292 (C)!", notifier=w157, error in (no error)=w156) -> ()  [unwired: 2 out]
          }
        }
        n75 = property on="Init PDA" class="Bool"("Disabled"=u8 2) -> ()  [unwired: 2 in, 2 out]
        n76 = property on="Init PDA" class="Bool"("Disabled"=w140) -> ()  [unwired: 2 in, 2 out]
      }
      event "Data Buffer Size": Value Change {
        n77 = event-data() -> ("NewVal"=w159:i16)  [unwired: 1 in]
        n78 = flat-sequence {
          tunnel: w159 -> [w160]
          frame #0 {
            n79 = global write "gGeneral.vi" "Buffer Size"(w160) -> ()
          }
          frame #1 {
            n80 = call "DataBuffer.vi"("Action"=T17."Resize Buffer") -> ()  [unwired: 10 in, 5 out]
          }
        }
      }
    }
    n81 = local read "Stop-All"() -> (w58:bool)
  }
  n82 = while "Data Sink 12" {
    tunnel: w31 -> [w167]
    tunnel: w30 -> [w169]
    shift-right: [w163] -> _
    shift-left: _ -> [w165]
    shift-left: _ -> [w164]
    stop <- w168 stop-if-true
    w162 = "\r"
    n83 = Wait on Notification(notifier=w167, error in (no error)=w169) -> (notification=w163:string, error out=w168:errorcluster)  [unwired: 2 in, 2 out]
    n84 = Concatenate Strings(w163, w162, w165, w162, w164, w162) -> (→"Status Message Board":string)
  }
  n85 = Obtain Notifier(name (unnamed)="Intensity Graph", notification data type=i32[][] array1024x30[30720 elements] ("Intensity Graph")) -> (notifier out=w27:refnum<notifier>, error out=w26:errorcluster)  [unwired: 2 in, 1 out]
  n86 = Obtain Notifier(name (unnamed)="Status", notification data type="" ("Status")) -> (notifier out=w18:refnum<notifier>, error out=w17:errorcluster)  [unwired: 2 in, 1 out]
  n87 = Obtain Notifier(name (unnamed)="PDA Temperature", notification data type=0.0) -> (notifier out=w9:refnum<notifier>, error out=w8:errorcluster)  [unwired: 2 in, 1 out]
  n88 = while {
    tunnel: w18 -> [w178]
    tunnel: w17 -> [w177]
    tunnel: w9 -> [w173]
    tunnel: w8 -> [w172]
    stop <- w170 stop-if-true
    n89 = Wait on Notification(notifier=w173, error in (no error)=w172) -> (notification=w171:dbl, error out=w170:errorcluster)  [unwired: 2 in, 2 out]
    "PDA Temperature" <- w171
    n90 = In Range and Coerce(upper limit=200.0, x=w171, lower limit=170.0) -> (In Range?=w174:bool)  [unwired: 1 out]
    n91 = case shown="False" w174 {
      tunnel: w178 -> [w181 _]
      tunnel: w177 -> [w180 _]
      frame False {
        n92 = Send Notification(notification="PDA Temperature out of range!!!", notifier=w181, error in (no error)=w180) -> ()  [unwired: 2 out]
      }
      frame True {
      }
    }
  }
  n93 = while {
    shift-right: [w187] -> _
    shift-left: _ -> [w188]
    shift-right: [w184] -> _
    shift-left: _ -> [w185]
    shift-right: [w183] -> _
    shift-left: _ -> [w182]
    stop <- FALSE stop-if-true
    n94 = event shown="[1] \"Ref Load\": Value Change" {
      selector: _ -> [_ _ _ _]
      dyn-events: _ -> [_ _ _ _]
      timeout: _ -> [_ _ _ _]
      tunnel: [w189 w196 w198 w201] -> w187
      tunnel: w188 -> [w191 w196 _ w201]
      tunnel: [w190 w194 w199 w202] -> w184
      tunnel: w185 -> [w190 w193 w199 w202]
      tunnel: [w189 w192 w200 w203] -> w183
      tunnel: w182 -> [_ w192 w200 w203]
      event "Batch Load": Value Change {
        n95 = event-data() -> ()  [unwired: 1 in, 1 out]
        n96 = call "Batch Load Data.vi"("Y Array Input"=w191) -> ("Data Array output"=w189:dbl[][])  [unwired: 8 in]
      }
      event "Ref Load": Value Change {
        n97 = event-data() -> ()  [unwired: 1 in, 1 out]
        n98 = call "Load Data.vi"("LoadData?"=TRUE, "Y-Array in"=w193) -> ("Y-Array out"=w194:dbl[])  [unwired: 3 in, 4 out]
      }
      event "Operation": Value Change {
        n99 = event-data() -> ()  [unwired: 1 in, 1 out]
        n100 = call "IntensityGraphOp_Dialog.vi"() -> ("Op-Mode output"=w197:T20)  [unwired: 2 in]
        "Op-Mode" <- w197
        n101 = call "IntensityGraphOperation.vi"("Op-Mode"=w197, "Ref Array"=w199, "Data Array"=w200) -> ("Data Array out"=w198:dbl[][])  [unwired: 2 in]
      }
      event "Print IntGraph": Value Change {
        n102 = event-data() -> ()  [unwired: 1 in, 1 out]
        n103 = call "Print IntGraph.vi"("Data IntGraph"=w201) -> ()  [unwired: 1 in]
      }
    }
    "Data IntGraph" <- w187
    "Waveform Graph" <- w184
  }
  n104 = while "Data Sink 14" {
    tunnel: w27 -> [w205]
    tunnel: w26 -> [w207]
    stop <- w206 stop-if-true
    n105 = Wait on Notification(notifier=w205, error in (no error)=w207) -> (notification=→"Intensity Graph":i32[][], error out=w206:errorcluster)  [unwired: 2 in, 2 out]
  }
  n106 = case shown="False" "Case Constant\n(See Context Help)" {
    frame False {
      w208 = FALSE ("Visible")
      n107 = property on="startCustSeq?" class="Bool"("Visible"=TRUE) -> ()  [unwired: 2 in, 2 out]
      n108 = property on="startSeq?" class="Bool"("Visible"=TRUE) -> ()  [unwired: 2 in, 2 out]
      n109 = property on="startCustSeq?" class="Bool"("Visible"=TRUE) -> ()  [unwired: 2 in, 2 out]
      n110 = property on="PauseCustSeq?" class="Bool (strict)"("Visible"=w208) -> ()  [unwired: 2 in, 2 out]
      n111 = property on="CancelCustSeq?" class="Bool (strict)"("Visible"=w208) -> ()  [unwired: 2 in, 2 out]
    }
    frame True {
      w212 = u8 2 ("Disabled")
      n112 = property on="startSeq?" class="Bool"("Disabled"=w212) -> ()  [unwired: 2 in, 2 out]
      n113 = property on="startCustSeq?" class="Bool"("Disabled"=w212) -> ()  [unwired: 2 in, 2 out]
      n114 = property on="nextShot" class="Bool"("Disabled"=w212) -> ()  [unwired: 2 in, 2 out]
    }
  }
  n115 = local read "FilePath_C"() -> (w3:T9)
  n116 = call "Get Shared Data Dir.vi"() -> ("Data Directory Path"=w2:path)  [unwired: 2 in, 1 out]
  n117 = Bundle By Name(cluster=w3, "Current Path"=w2) -> (w1:T9)
  n118 = Obtain Notifier(name (unnamed)="PDA Temperature", notification data type=0.0) -> (notifier out=w13:refnum<notifier>, error out=w12:errorcluster)  [unwired: 2 in, 1 out]
  n119 = local read "File Info"() -> (w53:T4)
  n120 = local write "FilePath_C"(w1) -> ()
  n121 = call "plotINIT.vi"("Plot Buffer Size"=u32 10) -> ("Pin"=w48:bool[], "Data Array output"=w46:dbl[][], "X-Axis Array output"=w47:dbl[][], "File Info Buffer Out"=w45:T4[])  [unwired: 1 out]
  n122 = Initialize Array(1300.0 ("element"), 1024 ("dimension size")) -> (w21:dbl[])
  n123 = Obtain Queue(name (unnamed)="File Info", element data type=w53) -> (queue out=w43:refnum<queue>, error out=w41:errorcluster)  [unwired: 3 in, 1 out]
  n124 = Obtain Queue(name (unnamed)="Y Data", element data type="Y Data") -> (queue out=w44:refnum<queue>, error out=w42:errorcluster)  [unwired: 3 in, 1 out]
  n125 = while "Main Loop" {
    shift-right: [w239] -> _
    shift-left: OpticsSS."Init" -> [w217]
    shift-right: [w234] -> _
    shift-left: w21 -> [w235]
    shift-right: [w233] -> _
    shift-left: _ -> [w232]
    shift-right: [w224] -> _
    shift-left: w21 -> [w225]
    shift-right: [w216] -> _
    shift-left: _ -> [w236]
    tunnel: w44 -> [w222]
    tunnel: w42 -> [w231]
    shift-right: [w230] -> _
    shift-left: w21 -> [w228]
    shift-right: [w229] -> _
    shift-left: _ -> [w226]
    tunnel: w43 -> [w223]
    tunnel: w41 -> [w227]
    tunnel: [w222] -> w52
    tunnel: [w223] -> w51
    tunnel: ["Master.vi" ("VI name")] -> w16
    tunnel: w13 -> [w214]
    tunnel: w12 -> [w213]
    stop <- w238 stop-if-true
    # "Need Sequence Parameters Register here"
    n126 = local read "FilePath_C"() -> (w221:T9)
    n127 = case shown="\"CCD_shot\"" w217 {
      tunnel: [OpticsSS."_Quit_" w265 w288 w393 w479 w506 w527 w555 w574 w590 w598 w624 OpticsSS."Ready" ("t")] -> w239
      tunnel: w236 -> [w240 _ w282 w400 w456 w513 w535 w558 w580 w588 w606 w627 w653]
      tunnel: [w240 w262 w283 w394 w478 w500 w534 w557 w579 w587 w602 w625 w653] -> w216
      tunnel: w235 -> [w243 w258 w287 w403 w470 w509 w538 w561 w583 w595 w608 w629 w656]
      tunnel: [w243 w258 w287 w403 w470 w509 w538 w561 w583 w595 w608 w611 w656] -> w234
      tunnel: [w242 w254 w286 w402 w472 w508 w537 w560 w582 w594 w607 w630 w655] -> w233
      tunnel: w232 -> [w242 w254 w286 w402 w472 w508 w537 w560 w582 w594 w607 w628 w655]
      tunnel: w222 -> [_ _ _ _ _ w514 _ _ _ _ _ w616 _]
      tunnel: w231 -> [_ _ _ _ _ _ _ _ _ _ _ w615 _]
      tunnel: [w244 w259 w284 w404 w477 w510 w539 w562 w584 w596 w609 w620 w657] -> w230
      tunnel: [w245 w260 w280 w392 w473 w498 w540 w563 w585 w597 w605 w613 w658] -> w229
      tunnel: w228 -> [w244 w259 w284 w404 _ w510 w539 w562 w584 w596 w609 w620 w657]
      tunnel: w223 -> [_ _ _ _ _ w511 _ _ _ _ _ w614 _]
      tunnel: w227 -> [_ _ _ _ _ _ _ _ _ _ _ _ _]
      tunnel: w226 -> [w245 w261 w281 w388 w457 w498 w540 w563 w585 w597 w605 w613 w658]
      tunnel: [w241 w257 w285 w401 w469 w507 w536 w559 w581 w593 w603 w610 w654] -> w224
      tunnel: w225 -> [w241 w257 w285 w401 w469 w507 w536 w559 w581 w593 w603 w618 w654]
      tunnel: w221 -> [_ _ _ w398 _ _ _ _ _ _ _ _ _]
      tunnel: "SubFolderNamesArray" -> [_ _ _ w399 _ _ _ _ _ _ _ _ _]
      tunnel: "HTL Array" -> [_ _ _ w397 _ _ _ _ _ _ _ _ _]
      tunnel: "Select Detector" -> [_ _ _ _ w465 _ _ _ _ w586 _ w617 _]
      tunnel: w214 -> [_ _ w279 _ _ _ _ _ _ _ _ _ _]
      tunnel: w213 -> [_ _ w278 _ _ _ _ _ _ _ _ _ _]
      frame "_Quit_" {
        # "The _Quit_ case has no corresponding state on the state diagram -\nit exists to indicate to the outer While Loop when to stop executing.\nThis case is executed immediately after the case for any terminal state, \nand is the last case to execute.  Place any general clean-up code here."
      }
      frame "Init" {
        (unwired) enum16{"err", "default"}."err"
        # "In initiation: disable inactive items\nbut do not pass it through \nerror cluster,\nor use special error handlers!"
        n128 = call "CCD_GPIB_Clear.vi"() -> ("error out"=w255:errorcluster)  [unwired: 5 in]
        n129 = call "FileInfo Updater.vi"("File Info"=w261) -> ("File Info output"=w264:T4)
        n130 = property on="Init PDA" class="Bool"("Disabled"=u8 0) -> ()  [unwired: 2 in, 2 out]
        n131 = property on="Init CCD" class="Bool"("Disabled"=u8 0) -> ()  [unwired: 2 in, 2 out]
        n132 = local read "CCD Parameters"() -> (w263:T7)
        n133 = flat-sequence {
          frame #0 {
            n134 = call "DataBuffer.vi"("Action"=T17."Initialize") -> ()  [unwired: 10 in, 5 out]
          }
          frame #1 {
            n135 = call "PlotSS.vi"("Mode"=PlottSS."Init") -> ()  [unwired: 11 in, 4 out]
          }
        }
        n136 = call "CCD_Initialization.vi"("error in"=w255, "Starting Action"=T14."Init GPIB") -> ("error out"=w262:errorcluster)  [unwired: 3 in, 4 out]
        n137 = Bundle By Name(cluster=w264, "CCD Parameters"=w263) -> (w260:T4)
        n138 = Obtain Notifier(name (unnamed)="Status", notification data type="" ("Status")) -> (notifier out=w251:refnum<notifier>, error out=w250:errorcluster)  [unwired: 2 in, 1 out]
        n139 = local write "File Info"(w260) -> ()
        n140 = case shown="No Error" w262 {
          tunnel: [OpticsSS."Ready" OpticsSS."Error Handler"] -> w265
          tunnel: w251 -> [w271 w275]
          tunnel: w250 -> [w270 w274]
          frame No Error {
            w269 = u8 0 ("Disabled")
            n141 = property on="startSeq?" class="Bool"("Disabled"=w269) -> ()  [unwired: 2 in, 2 out]
            n142 = property on="startCustSeq?" class="Bool"("Disabled"=w269) -> ()  [unwired: 2 in, 2 out]
            n143 = property on="nextShot" class="Bool"("Disabled"=w269, "Blinking"=FALSE) -> ()  [unwired: 2 in, 2 out]
            n144 = Send Notification(notification="Welcome to NHMFL", notifier=w271, error in (no error)=w270) -> ()  [unwired: 2 out]
          }
          frame Error {
            n145 = Send Notification(notification="Call Xing Wei @ 4-1060 (O), or 668-0504 (H), or 591-6292 (C)!", notifier=w275, error in (no error)=w274) -> ()  [unwired: 2 out]
          }
        }
        n146 = local write "Stop-All"(FALSE ("Stop-All")) -> ()
      }
      frame "Ready" {
        n147 = while {
          tunnel: [w296] -> w288
          shift-right: [w291] -> w283
          shift-left: w282 -> [w291]
          shift-right: [w293] -> w280
          shift-left: w281 -> [w292]
          tunnel: w279 -> [w290]
          tunnel: w278 -> [w289]
          stop <- w295 stop-if-true
          n148 = event shown="[0] Timeout" {
            selector: _ -> [_ _ _ _ _ _ _ _]
            dyn-events: _ -> [_ _ _ _ _ _ _ _]
            timeout: 500 -> [_ _ _ _ _ _ _ _]
            tunnel: [w310 OpticsSS."HTL" OpticsSS."BG_Setup" w350 OpticsSS."HTL" OpticsSS."CCDSetup" OpticsSS."Calibration" OpticsSS."Ready" ("f")] -> w296
            tunnel: [w299 TRUE TRUE TRUE w361 TRUE TRUE _] -> w295
            tunnel: [w312 w327 w331 w342 w370 w373 w376 w382] -> w293
            tunnel: w292 -> [_ w328 w331 w344 w371 w373 w376 w382]
            tunnel: w290 -> [w298 _ _ _ _ _ _ _]
            tunnel: w289 -> [w297 _ _ _ _ _ _ _]
            event Timeout {
              w301 = T3 0 items=["N.A.", "OK", "Busy", "Done"] ("y")
              w303 = T3 0 items=["N.A.", "OK", "Busy", "Done"] ("y")
              w306 = OperationMode.ctt."Standby" ("Operation Mode")
              n149 = event-data() -> ()  [unwired: 1 in, 2 out]
              n150 = global read "gStatus.vi" "PDA"() -> (w302:T3)
              n151 = local read "File Info"() -> (w308:T4)
              n152 = Not Equal?(x=w302, y=w301) -> (x != y?=w300:bool)
              "InGaAs OK?" <- w300
              n153 = global read "gStatus.vi" "CCD"() -> (w305:T3)
              n154 = Bundle By Name(cluster=w308, "Operation Mode"=w306) -> (w307:T4)
              n155 = local write "Operation Mode"(w306) -> ()
              n156 = property on="PDA Temperature" class="WFChart (strict)"("Visible"=w300) -> ()  [unwired: 2 in, 2 out]
              n157 = call "CheckAll-Quit.vi"() -> ("All-Quit"=w299:bool)  [unwired: 3 in]
              n158 = Not Equal?(x=w305, y=w303) -> (x != y?=→"CCD OK?":bool)
              n159 = case shown="True" w300 {
                selector: w300 -> [_ w316]
                tunnel: w298 -> [_ w315]
                tunnel: w297 -> [_ w314]
                frame False {
                }
                frame True {
                  n160 = call "PDA_Temperature_Readout.vi"("stop"=w316, "msec to wait"=u32 0) -> ("PDA Temperature"=w313:dbl)  [unwired: 4 in, 1 out]
                  n161 = Send Notification(notification=w313, notifier=w315, error in (no error)=w314) -> ()  [unwired: 2 out]
                }
              }
              n162 = Select(t=OpticsSS."_Quit_", s=w299, f=OpticsSS."Ready") -> (s? t:f=w310:T1)
              n163 = call "FileInfo Updater.vi"("File Info"=w307) -> ("File Info output"=w312:T4)
            }
            event "nextShot": Value Change {
              w326 = OperationMode.ctt."CCD Single Shot" ("Operation Mode")
              n164 = event-data() -> ()  [unwired: 1 in, 1 out]
              n165 = property on="nextShot" class="Bool"("Disabled"=u8 2, "Blinking"=TRUE) -> ()  [unwired: 2 in, 2 out]
              n166 = local write "Operation Mode"(w326) -> ()
              n167 = Bundle By Name(cluster=w328, "Index_repetition"=u16 0, "Operation Mode"=w326) -> (w327:T4)
              n168 = Obtain Notifier(name (unnamed)="Experiment Running", notification data type=FALSE ("SaveData?")) -> (notifier out=w322:refnum<notifier>, error out=w323:errorcluster)  [unwired: 2 in, 1 out]
              n169 = Send Notification(notification=TRUE, notifier=w322, error in (no error)=w323) -> ()  [unwired: 2 out]
            }
            event "BkgrdShot": Value Change {
              n170 = event-data() -> ()  [unwired: 1 in, 1 out]
            }
            event "startSeq?": Value Change {
              w343 = OperationMode.ctt."CCD Sequence Shots" ("Operation Mode")
              n171 = local read "FilePath_C"() -> (w337:T9)
              n172 = event-data() -> ()  [unwired: 1 in, 1 out]
              n173 = local write "Operation Mode"(w343) -> ()
              n174 = call "Paths_for_Seq_Shot.vi"("File Path"=w337, "FieldRamp Parameters"="HRamp Paras", "RampIndexSelect"="RampSelect") -> ("File Path Para Array out"=w335:T9[], "FieldRamp Parameters out"=w349:dbl[][], "RampIndexSelect out"=w348:bool[])  [unwired: 2 in]
              n175 = local write "HRamp Paras"(w349) -> ()
              n176 = Or Array Elements(Boolean array=w348) -> (logical OR=w336:bool)
              n177 = case shown="True" w336 {
                tunnel: [OpticsSS."Ready" ("f") OpticsSS."HTL"] -> w350
                frame False {
                }
                frame True {
                  n178 = property on="startSeq?" class="Bool"("Visible"=FALSE) -> ()  [unwired: 2 in, 2 out]
                  n179 = Obtain Notifier(name (unnamed)="Experiment Running", notification data type=FALSE ("SaveData?")) -> (notifier out=w355:refnum<notifier>, error out=w354:errorcluster)  [unwired: 2 in, 1 out]
                  n180 = Send Notification(notification=TRUE, notifier=w355, error in (no error)=w354) -> ()  [unwired: 2 out]
                }
              }
              n181 = call "HTL parameters.vi"("Move on"=TRUE, "Tab Control"=enum32{"Fixed Steps", "Free Style Steps"}."Fixed Steps", "RampSelect"=w348, "File Path Para Array"=w335, "FieldRamp Parameters"=w349) -> ("HTL Array"=w345:dbl[][], "Path array"=→"Path array":path[])  [unwired: 3 in, 2 out]
              n182 = Bundle By Name(cluster=w344, "Index_repetition"=u16 0, "Index"=u16 1, "Operation Mode"=w343) -> (w342:T4)
              n183 = property on="PauseSeq?" class="Bool (strict)"("Visible"=w336) -> ()  [unwired: 2 in, 2 out]
              n184 = property on="CancelSeq?" class="Bool (strict)"("Visible"=w336) -> ()  [unwired: 2 in, 2 out]
              n185 = local write "HTL Array"(w345) -> ()
            }
            event "startCustSeq?": Value Change {
              w369 = OperationMode.ctt."CCD Custom Shots" ("Operation Mode")
              w361 = TRUE
              n186 = event-data() -> ()  [unwired: 1 in, 1 out]
              n187 = property on="startCustSeq?" class="Bool"("Visible"=FALSE) -> ()  [unwired: 2 in, 2 out]
              n188 = local write "Operation Mode"(w369) -> ()
              n189 = Bundle By Name(cluster=w371, "Index_repetition"=u16 0, "Index"=u16 1, "Operation Mode"=w369) -> (w370:T4)
              n190 = Obtain Notifier(name (unnamed)="Experiment Running", notification data type=FALSE ("SaveData?")) -> (notifier out=w364:refnum<notifier>, error out=w363:errorcluster)  [unwired: 2 in, 1 out]
              n191 = property on="CancelCustSeq?" class="Bool (strict)"("Visible"=w361) -> ()  [unwired: 2 in, 2 out]
              n192 = property on="PauseCustSeq?" class="Bool (strict)"("Visible"=w361) -> ()  [unwired: 2 in, 2 out]
              n193 = Send Notification(notification=TRUE, notifier=w364, error in (no error)=w363) -> ()  [unwired: 2 out]
            }
            event "CCD LineSet?": Value Change {
              n194 = event-data() -> ()  [unwired: 1 in, 1 out]
            }
            event "Calibration": Value Change {
              n195 = event-data() -> ()  [unwired: 1 in, 1 out]
            }
            event "Cust Seq Para Setup": Value Change {
              n196 = event-data() -> ()  [unwired: 1 in, 1 out]
              n197 = local read "HRamp Paras"() -> (w380:dbl[][])
              n198 = local read "RampSelect"() -> (w381:bool[])
              n199 = call "HTL parameters.vi"("RampSelect"=w381, "FieldRamp Parameters"=w380) -> ("HTL Array"=w384:dbl[][], "Prefix Indexed output"=w379:bool, "SubFolderNamesArray"=w383:string[])  [unwired: 6 in, 1 out]
              n200 = local write "HTL Array"(w384) -> ()
              n201 = local write "SubFolderNamesArray"(w383) -> ()
              n202 = local write "Prefix_indexed"(w379) -> ()
            }
          }
        }
      }
      frame "HTL" {
        n203 = local read "Path array"() -> (w390:path[])
        n204 = local read "File Info"() -> (w389:T4)
        n205 = Unbundle By Name(w389) -> ("CCD Parameters"=w386:T7)
        n206 = Bundle By Name(cluster=w388, "CCD Parameters"=w386) -> (w387:T4)
        n207 = call "ith HTL.vi"("HTL Array"=w397, "File Info input"=w387, "Prefix Indexed"="Prefix_indexed", "SubFolderNamesArray"=w399, "error in"=w400, "Path array"=w390, "File Path Parameter"=w398) -> ("Stop?"=w396:bool, "File Info output"=w392:T4, "error out"=w395:errorcluster)  [unwired: 6 in]
        n208 = case shown="True" w396 {
          tunnel: [w409 w428] -> w394
          tunnel: w395 -> [w409 w429]
          tunnel: [w405 w425] -> w393
          tunnel: w392 -> [w411 w431]
          frame False {
            n209 = Unbundle By Name(w411) -> ("CCD Parameters.dt or s"=w412:dbl)
            n210 = Unbundle By Name(w409) -> ("status"=w416:bool)
            n211 = while {
              tunnel: [w417] -> w408
              stop <- w419 continue-if-true
              n212 = call "CheckCancel.vi"() -> ("Cancelled"=w417:bool)  [unwired: 2 in, 1 out]
              n213 = Not(x=w417) -> (.not. x?=w421:bool)
              n214 = Wait Until Next ms Multiple(millisecond multiple=u32 100) -> ()  [unwired: 1 out]
              n215 = Or(x="PauseCustSeq?", y="PauseSeq?") -> (x .or. y?=w420:bool)
              n216 = And(x=w420, y=w421) -> (x .and. y?=w419:bool)
            }
            n217 = Select(t=OpticsSS."HTL Error", s=w416, f=OpticsSS."CCD_shot") -> (s? t:f=w406:T1)
            n218 = Multiply(x=w412, y=1000.0) -> (x*y=w413:dbl)
            n219 = Wait (ms)(milliseconds to wait=w413) -> ()  [unwired: 1 out]
            n220 = Select(t=OpticsSS."Error Handler", s=w408, f=w406) -> (s? t:f=w405:T1)
          }
          frame True {
            n221 = Unbundle By Name(w431) -> ("Operation Mode"=w430:T2)
            n222 = case shown="\"CCD Single Shot\", Default" w430 {
              tunnel: w429 -> [w434 w439 w446]
              tunnel: [w434 w438 w447] -> w428
              frame "CCD Single Shot", Default {
                n223 = property on="nextShot" class="Bool"("Disabled"=u8 0, "Blinking"=FALSE) -> ()  [unwired: 2 in, 2 out]
              }
              frame "CCD Sequence Shots" {
                w435 = FALSE ("Visible")
                n224 = case shown="True" "Park Seq" {
                  tunnel: w439 -> [w440 w443]
                  tunnel: [w440 w442] -> w438
                  frame False {
                  }
                  frame True {
                    n225 = call "PS Control Write.vi"("Ramp"=FALSE, "error in (no error)"=w443) -> ("error out"=w442:errorcluster)  [unwired: 12 in, 1 out]
                  }
                }
                n226 = property on="startSeq?" class="Bool"("Visible"=TRUE) -> ()  [unwired: 2 in, 2 out]
                n227 = property on="PauseSeq?" class="Bool (strict)"("Visible"=w435) -> ()  [unwired: 2 in, 2 out]
                n228 = property on="CancelSeq?" class="Bool (strict)"("Visible"=w435) -> ()  [unwired: 2 in, 2 out]
              }
              frame "CCD Custom Shots" {
                w445 = FALSE ("Visible")
                n229 = property on="startCustSeq?" class="Bool"("Visible"=TRUE) -> ()  [unwired: 2 in, 2 out]
                n230 = property on="PauseCustSeq?" class="Bool (strict)"("Visible"=w445) -> ()  [unwired: 2 in, 2 out]
                n231 = property on="CancelCustSeq?" class="Bool (strict)"("Visible"=w445) -> ()  [unwired: 2 in, 2 out]
                n232 = case shown="True" "Park Cust Seq" {
                  tunnel: w446 -> [w449 w452]
                  tunnel: [w449 w451] -> w447
                  frame False {
                  }
                  frame True {
                    n233 = call "PS Control Write.vi"("Ramp"=FALSE, "error in (no error)"=w452) -> ("error out"=w451:errorcluster)  [unwired: 12 in, 1 out]
                  }
                }
              }
            }
            n234 = call "CheckCancel.vi"() -> ("Cancelled"=w427:bool)  [unwired: 2 in, 1 out]
            n235 = Select(t=OpticsSS."Error Handler", s=w427, f=OpticsSS."Ready") -> (s? t:f=w425:T1)
          }
        }
      }
      frame "CCD_shot" {
        n236 = Unbundle By Name(w457) -> ("CCD Parameters"=w466:T7, "Exp Index"=w475:u32)
        n237 = global read "gHField.vi" "PS Current"() -> (w454:dbl)
        n238 = Obtain Notifier(name (unnamed)="Status", notification data type="" ("Status")) -> (notifier out=w460:refnum<notifier>, error out=w459:errorcluster)  [unwired: 2 in, 1 out]
        n239 = flat-sequence {
          tunnel: [w481] -> w455
          tunnel: w456 -> [w481]
          tunnel: [w480] -> w453
          tunnel: w454 -> [w480]
          frame #0 {
          }
        }
        n240 = Increment(x=w475) -> (x+1=w474:u32)
        n241 = call "CCD-PDA_Exposure.vi"("Current Detector"=w465, "error in"=w455, "CCD Parameters"=w466) -> ("Error Out"=w468:errorcluster, "The Data"=w471:dbl[], "#PixelOverflow"=→"#PixelOverflow":u32, "PixelOverflow"=w463:bool)  [unwired: 2 in]
        "Pixel Overflow" <- w463
        n242 = Send Notification(notification="Taking Data!", notifier=w460, error in (no error)=w459) -> ()  [unwired: 2 out]
        n243 = global write "gStatus.vi" "Exp Index"(w474) -> ()
        n244 = Bundle By Name(cluster=w457, "Exp Index"=w474, "Field (T)"=w453) -> (w473:T4)
        n245 = call "CCD-PDA_ExposureTime.vi"("Current Detector"=w465, "CCD Parameters"=w466) -> ("Exposure Time (s)"=w464:dbl)  [unwired: 2 in]
        n246 = property on="Pixel Overflow" class="Bool (strict)"("Visible"=w463, "Blinking"=w463) -> ()  [unwired: 2 in, 2 out]
        n247 = property on="#PixelOverflow" class="DigNum (strict)"("Visible"=w463) -> ()  [unwired: 2 in, 2 out]
        n248 = call "CCD-PDA_Background_Correct.vi"("Operation Mode"=w472, "Select Detector"=w465, "The InGaAs PDA FPN in"=w469, "The Reference Data In"=w470, "CCD Parameters"=w466, "The Signal Data In"=w471) -> ("The Signal Data Out"=w477:dbl[])  [unwired: 3 in]
        n249 = case shown="No Error" w468 {
          selector: w468 -> [w483 w491]
          tunnel: [OpticsSS."QueueData" w486] -> w479
          tunnel: [w483 w490] -> w478
          frame No Error {
            n250 = property on="Exposure time display" class="Slide (strict)"("Visible"=FALSE) -> ()  [unwired: 2 in, 2 out]
          }
          frame Error {
            n251 = call "CheckCancel.vi"("error in (no error)"=w491) -> ("Cancelled"=w488:bool, "error out"=w490:errorcluster)  [unwired: 1 in]
            n252 = property on="Exposure time display" class="Slide (strict)"("Visible"=FALSE) -> ()  [unwired: 2 in, 2 out]
            n253 = Select(t=OpticsSS."Error Handler", s=w488, f=OpticsSS."CCD Error") -> (s? t:f=w486:T1)
          }
        }
        n254 = property on="Exposure time display" class="Slide (strict)"("Visible"=TRUE, "Scale.Range:Maximum"=w464) -> ()  [unwired: 2 in, 2 out]
        n255 = local write "ExpTimeTarget"(w464) -> ()
      }
      frame "QueueData" {
        n256 = global read "gHField.vi" "PS Current"() -> (w496:dbl)
        n257 = Unbundle By Name(w498) -> ("Field (T)"=w495:dbl)
        n258 = Enqueue Element(queue=w514, element=w510, error in (no error)=w513) -> (error out=w512:errorcluster)  [unwired: 1 in, 2 out]
        n259 = Or(x="CancelSeq?", y="CancelCustSeq?") -> (x .or. y?=w502:bool)
        n260 = Add(x=w496, y=w495) -> (x+y=w494:dbl)
        n261 = Divide(x=w494, y=2.0) -> (x/y=w493:dbl)
        n262 = Bundle By Name(cluster=w498, "Field (T)"=w493) -> (w497:T4)
        n263 = Enqueue Element(queue=w511, element=w497, error in (no error)=w512) -> (error out=w501:errorcluster)  [unwired: 1 in, 2 out]
        n264 = call "CheckCancel.vi"("error in (no error)"=w501) -> ("Cancelled"=w499:bool, "error out"=w500:errorcluster)  [unwired: 1 in]
        n265 = Or(x=w499, y=w502) -> (x .or. y?=w503:bool)
        n266 = case shown="True" w503 {
          tunnel: [OpticsSS."HTL" ("t") w517] -> w506
          tunnel: w499 -> [_ w519]
          frame False {
          }
          frame True {
            w520 = FALSE ("Blinking")
            w521 = TRUE ("Visible")
            w524 = FALSE ("CancelSeq?")
            n267 = property on="startCustSeq?" class="Bool"("Visible"=w521) -> ()  [unwired: 2 in, 2 out]
            n268 = property on="startSeq?" class="Bool"("Visible"=w521) -> ()  [unwired: 2 in, 2 out]
            n269 = property on="PauseCustSeq?" class="Bool (strict)"("Visible"=w520) -> ()  [unwired: 2 in, 2 out]
            n270 = property on="PauseSeq?" class="Bool (strict)"("Visible"=w520) -> ()  [unwired: 2 in, 2 out]
            n271 = property on="CancelSeq?" class="Bool (strict)"("Visible"=w520) -> ()  [unwired: 2 in, 2 out]
            n272 = property on="CancelCustSeq?" class="Bool (strict)"("Visible"=w520) -> ()  [unwired: 2 in, 2 out]
            n273 = Select(t=OpticsSS."Error Handler", s=w519, f=OpticsSS."Ready" ("t")) -> (s? t:f=w517:T1)
            n274 = local write "CancelCustSeq?"(w524) -> ()
            n275 = local write "CancelSeq?"(w524) -> ()
            n276 = property on="nextShot" class="Bool"("Disabled"=u8 0, "Blinking"=FALSE) -> ()  [unwired: 2 in, 2 out]
          }
        }
      }
      frame "Error Handler" {
        n277 = call "General_ErrorHandler.vi"("error in"=w535) -> ("error out"=w534:errorcluster, "All-Quit"=w529:bool)  [unwired: 5 in, 1 out]
        n278 = Obtain Notifier(name (unnamed)="Status", notification data type="" ("Status")) -> (notifier out=w531:refnum<notifier>, error out=w530:errorcluster)  [unwired: 2 in, 1 out]
        n279 = case shown="No Error" w534 {
          tunnel: [OpticsSS."Ready" OpticsSS."_Quit_"] -> w528
          tunnel: w531 -> [_ w551]
          tunnel: w530 -> [_ w550]
          frame No Error {
            w547 = u8 0 ("Disabled")
            w542 = FALSE ("Visible")
            w543 = FALSE ("Visible")
            w544 = TRUE ("Visible")
            n280 = property on="startSeq?" class="Bool"("Disabled"=w547, "Visible"=w544) -> ()  [unwired: 2 in, 2 out]
            n281 = property on="startCustSeq?" class="Bool"("Disabled"=w547, "Visible"=w544) -> ()  [unwired: 2 in, 2 out]
            n282 = property on="nextShot" class="Bool"("Disabled"=w547, "Visible"=w544, "Blinking"=FALSE) -> ()  [unwired: 2 in, 2 out]
            n283 = property on="Init PDA" class="Bool"("Disabled"=u8 0) -> ()  [unwired: 2 in, 2 out]
            n284 = property on="Init CCD" class="Bool"("Disabled"=u8 0) -> ()  [unwired: 2 in, 2 out]
            n285 = property on="PauseCustSeq?" class="Bool (strict)"("Visible"=w542) -> ()  [unwired: 2 in, 2 out]
            n286 = property on="CancelCustSeq?" class="Bool (strict)"("Visible"=w542) -> ()  [unwired: 2 in, 2 out]
            n287 = property on="PauseSeq?" class="Bool (strict)"("Visible"=w543) -> ()  [unwired: 2 in, 2 out]
            n288 = property on="CancelSeq?" class="Bool (strict)"("Visible"=w543) -> ()  [unwired: 2 in, 2 out]
          }
          frame Error {
            n289 = Send Notification(notification="Fatal Error!!!!!\nCall Xing Wei @ 4-1060 (O), or 668-0504 (H), or 591-6292 (C)!", notifier=w551, error in (no error)=w550) -> ()  [unwired: 2 out]
          }
        }
        n290 = property on="Exposure time display" class="Slide (strict)"("Visible"=FALSE) -> ()  [unwired: 2 in, 2 out]
        n291 = Select(t=OpticsSS."_Quit_", s=w529, f=w528) -> (s? t:f=w527:T1)
      }
      frame "HTL Error" {
        n292 = call "HTL_ErrorHandler.vi"("error in"=w558) -> ("error out"=w557:errorcluster, "All-Quit"=w554:bool)  [unwired: 6 in]
        n293 = case shown="Error" w557 {
          tunnel: [OpticsSS."CCD_shot" OpticsSS."Error Handler"] -> w556
          frame No Error {
          }
          frame Error {
            w565 = FALSE ("Visible")
            w568 = FALSE ("Visible")
            n294 = property on="nextShot" class="Bool"("Disabled"=u8 0, "Blinking"=FALSE) -> ()  [unwired: 2 in, 2 out]
            n295 = property on="startCustSeq?" class="Bool"("Visible"=TRUE) -> ()  [unwired: 2 in, 2 out]
            n296 = property on="startSeq?" class="Bool"("Visible"=TRUE) -> ()  [unwired: 2 in, 2 out]
            n297 = property on="PauseSeq?" class="Bool (strict)"("Visible"=w565) -> ()  [unwired: 2 in, 2 out]
            n298 = property on="CancelSeq?" class="Bool (strict)"("Visible"=w565) -> ()  [unwired: 2 in, 2 out]
            n299 = property on="PauseCustSeq?" class="Bool (strict)"("Visible"=w568) -> ()  [unwired: 2 in, 2 out]
            n300 = property on="CancelCustSeq?" class="Bool (strict)"("Visible"=w568) -> ()  [unwired: 2 in, 2 out]
          }
        }
        n301 = Select(t=OpticsSS."_Quit_", s=w554, f=w556) -> (s? t:f=w555:T1)
      }
      frame "CCD Error" {
        n302 = call "CCD_PDA_ErrorHandler.vi"("error in"=w580) -> ("error out"=w579:errorcluster, "All-Quit"=w573:bool)  [unwired: 6 in]
        n303 = Unbundle By Name(w579) -> ("status"=w578:bool)
        n304 = Select(t=OpticsSS."Error Handler", s=w578, f=OpticsSS."CCD_shot") -> (s? t:f=w575:T1)
        n305 = Select(t=OpticsSS."_Quit_", s=w573, f=w575) -> (s? t:f=w574:T1)
      }
      frame "CCDSetup" {
        n306 = call "Detector_setup.vi"("Select Detector"=w586, "error in"=w588) -> ("error out"=w587:errorcluster)  [unwired: 6 in]
        n307 = Unbundle By Name(w587) -> ("status"=w592:bool)
        n308 = Select(t=OpticsSS."Error Handler", s=w592, f=OpticsSS."Ready") -> (s? t:f=w590:T1)
      }
      frame "Calibration" {
        n309 = call "FileInfo Updater.vi"("File Info"=w605) -> ("File Info output"=w604:T4)
        n310 = call "McP Calibrate.vi"("File Info In"=w604, "error in"=w606) -> ("error out"=w602:errorcluster)  [unwired: 13 in]
        n311 = Unbundle By Name(w602) -> ("status"=w601:bool)
        n312 = Select(t=OpticsSS."Error Handler", s=w601, f=OpticsSS."Ready") -> (s? t:f=w598:T1)
      }
      frame "BG_Setup" {
        n313 = Unbundle By Name(w613) -> ("CCD Parameters"=w619:T7)
        n314 = call "CCD-PDA_Background_Setup.vi"("The Reference Data In"=w629, "CCD Parameters"=w619, "Operation Mode"=w628, "PDA Fixed Pattern (FPN) Data In"=w618, "error in"=w627, "Current Detector"=w617) -> ("The Reference Data Out"=w611:dbl[], "Operation Output"=w630:u8, "PDA Fixed Pattern (FPN) Data Out"=w610:dbl[], "Reference Type output"=w623:T22, "PDA-FPN Setup out"=w612:bool, "Error Out"=w626:errorcluster)  [unwired: 4 in]
        n315 = Equal?(x=w623, y=T22."The Reference CCD Shot") -> (x = y?=w621:bool)
        n316 = case shown="Error" w626 {
          selector: w626 -> [w640 w651]
          tunnel: [w640 w651] -> w625
          tunnel: [OpticsSS."Ready" OpticsSS."Error Handler"] -> w624
          tunnel: w621 -> [w638 _]
          tunnel: w616 -> [w637 _]
          tunnel: w615 -> [w636 _]
          tunnel: w614 -> [w635 _]
          tunnel: w613 -> [w634 _]
          tunnel: w612 -> [w633 _]
          tunnel: w611 -> [w632 _]
          tunnel: w610 -> [w631 _]
          frame No Error {
            n317 = case shown="True" w638 {
              tunnel: w637 -> [_ w648]
              tunnel: w636 -> [_ w647]
              tunnel: w635 -> [_ w646]
              tunnel: w634 -> [_ w645]
              tunnel: w633 -> [_ w644]
              tunnel: w632 -> [_ w642]
              tunnel: w631 -> [_ w643]
              frame False {
              }
              frame True {
                n318 = Select(t=w643, s=w644, f=w642) -> (s? t:f=w641:dbl[])
                n319 = Enqueue Element(queue=w648, element=w641, error in (no error)=w647) -> (error out=w649:errorcluster)  [unwired: 1 in, 2 out]
                n320 = Enqueue Element(queue=w646, element=w645, error in (no error)=w649) -> ()  [unwired: 1 in, 3 out]
              }
            }
          }
          frame Error {
          }
        }
      }
      frame "HTL Paras Setup" {
        # "Maybe I do not need to have this case."
      }
    }
    "Error" <- w216
    n321 = Equal?(x=w217, y=OpticsSS."_Quit_") -> (x = y?=w238:bool)
    "Master State" <- w217
  }
  n322 = Obtain Queue(max queue size (-1, unlimited)=1, name (unnamed)="OddReady", element data type=FALSE ("Boolean")) -> (queue out=w5:refnum<queue>)  [unwired: 2 in, 2 out]
  n323 = while {
    shift-right: [w689] -> _
    shift-left: w47 -> [w692]
    shift-right: [w688] -> _
    shift-left: w46 -> [w691]
    shift-right: [w673] -> _
    shift-left: w45 -> [w690]
    shift-right: [w677] -> _
    shift-left: w48 -> [w682]
    shift-right: [w672] -> _
    shift-left: _ -> [w671]
    shift-right: [w669] -> _
    shift-left: _ -> [w667]
    shift-right: [w668] -> _
    shift-left: _ -> [w666]
    tunnel: w44 -> [w665]
    tunnel: w43 -> [w664]
    tunnel: w42 -> [w663]
    tunnel: w41 -> [w662]
    tunnel: w5 -> [w659]
    stop <- w660 stop-if-true
    n324 = event shown="[0] Timeout" {
      selector: _ -> [_ _ _ _ _ _ _ _ _]
      dyn-events: _ -> [_ _ _ _ _ _ _ _ _]
      timeout: 100 -> [_ _ _ _ _ _ _ _ _]
      tunnel: w692 -> [w698 w788 w800 w814 w825 w837 w863 w914 w924]
      tunnel: w691 -> [w697 w787 w799 w813 w824 w836 w862 w913 w923]
      tunnel: w690 -> [w694 w786 w798 w812 w823 w835 w869 w912 w922]
      tunnel: [w700 w784 w800 w814 w825 w837 w863 w914 w924] -> w686
      tunnel: [w699 w783 w799 w813 w824 w836 w862 w913 w923] -> w685
      tunnel: [w695 w782 w798 w812 w823 w835 w869 w912 w922] -> w687
      tunnel: [w696 PlottSS."load" ("Mode") PlottSS."Trace-Show/Hide" ("Mode") PlottSS."Pin-Mix" ("Mode") PlottSS."Unit-Change" ("Mode") PlottSS."Column Heading" ("Mode") PlottSS."_Quit_" ("Mode") PlottSS."_Quit_" ("Mode") PlottSS."Display/Print" ("Mode")] -> w684
      tunnel: [w722 w780 w797 w802 w821 w833 w867 w910 w920] -> w677
      tunnel: [_ _ _ w810 _ _ _ _ _] -> w683
      tunnel: w682 -> [w722 w780 w797 w806 w821 w833 w867 w910 w920]
      tunnel: [w720 w779 w792 w807 w819 w831 w866 w909 w918] -> w681
      tunnel: "Trace" -> [w720 w779 _ w807 w819 w831 w866 w909 w918]
      tunnel: [w719 w778 w796 w808 w820 w832 w865 w908 w915] -> w680
      tunnel: "Print?" -> [w719 w778 w796 w808 w820 w832 w865 w908 _]
      tunnel: [w721 w777 w795 w809 w818 w830 w857 w880 w919] -> w679
      tunnel: "X-Axis Unit" -> [w721 w777 w795 w809 _ w830 w857 w880 w919]
      tunnel: "Column Headings" -> [_ _ _ w805 _ _ _ _ _]
      tunnel: [w718 _ _ _ _ w828 w864 w907 _] -> w670
      tunnel: w671 -> [w718 _ _ _ _ w828 w864 w907 _]
      tunnel: [w717 w776 w794 w804 w816 w827 w843 w884 w917] -> w669
      tunnel: [w716 w775 w793 w803 w815 w826 w842 w883 w916] -> w668
      tunnel: w667 -> [w717 w776 w794 w804 w816 w827 w841 w884 w917]
      tunnel: w666 -> [w716 w775 w793 w803 w815 w826 w840 w883 w916]
      tunnel: w665 -> [w715 _ _ _ _ _ _ _ _]
      tunnel: w664 -> [w714 _ _ _ _ _ _ _ _]
      tunnel: w663 -> [w704 _ _ _ _ _ _ _ _]
      tunnel: w662 -> [w703 _ _ _ _ _ _ _ _]
      tunnel: w659 -> [w693 _ _ _ _ _ _ _ _]
      event Timeout {
        n325 = event-data() -> ()  [unwired: 1 in, 1 out]
        n326 = Get Queue Status(queue=w715, error in (no error)=w704) -> (queue out=w706:refnum<queue>, error out=w702:errorcluster, # elements in queue=w713:i32)  [unwired: 1 in, 5 out]
        n327 = Get Queue Status(queue=w714, error in (no error)=w703) -> (queue out=w705:refnum<queue>, error out=w701:errorcluster, # elements in queue=w710:i32)  [unwired: 1 in, 5 out]
        n328 = Greater?(x=w710, y=0) -> (0:w708:bool)
        n329 = Greater?(x=w713, y=0) -> (0:w709:bool)
        n330 = And(x=w709, y=w708) -> (x .and. y?=w707:bool)
        n331 = case shown="True" w707 {
          tunnel: w706 -> [_ w758]
          tunnel: w705 -> [_ w757]
          tunnel: w702 -> [_ w756]
          tunnel: w701 -> [_ w755]
          tunnel: [w735 w749] -> w700
          tunnel: [w734 w748] -> w699
          tunnel: w698 -> [w735 _]
          tunnel: w697 -> [w734 _]
          tunnel: [PlottSS."_Quit_" ("Mode") PlottSS."load" ("Mode")] -> w696
          tunnel: [w732 w746] -> w695
          tunnel: w694 -> [w732 _]
          tunnel: w693 -> [_ w737]
          frame False {
          }
          frame True {
            # "Need Plot buffer size here"
            n332 = local read "Operation Mode"() -> (w743:T2)
            n333 = Dequeue Element(queue=w758, error in (no error)=w756) -> (element=w753:dbl[])  [unwired: 1 in, 3 out]
            n334 = Dequeue Element(queue=w757, error in (no error)=w755) -> (element=w754:T4)  [unwired: 1 in, 3 out]
            n335 = case shown="\"CCD Sequence Shots\"" w743 {
              tunnel: [_ _ TRUE TRUE _ _ _ _] -> w742
              frame "Standby", Default {
              }
              frame "CCD Single Shot" {
              }
              frame "CCD Sequence Shots" {
              }
              frame "CCD Custom Shots" {
              }
              frame "CCD Reference Shot" {
              }
              frame "Step Scanning " {
              }
              frame "Time Scanning" {
              }
              frame "NML Data Acquisition" {
              }
            }
            n336 = Or(x="AutoSaveData", y=w742) -> (x .or. y?=w745:bool)
            n337 = case shown="True" w745 {
              tunnel: w754 -> [w766 w770]
              tunnel: w753 -> [w765 w768]
              tunnel: [w766 w769] -> w741
              tunnel: [w765 w768] -> w752
              frame False {
              }
              frame True {
                n338 = call "Save Data.vi"("FileFormat"="File Format", "Saving Mode"=T23."Auto Data Saving", "Data"=w768, "File Info Input"=w770, "User Comments"="User Comments", "File Parameter"="FilePath_C") -> ("File Info output"=w769:T4)  [unwired: 5 in]
                n339 = Unbundle By Name(w769) -> ("FilePath"=→"Most recently saved file":path)
              }
            }
            n340 = call "DataBuffer.vi"("File Info In"=w741, "Action"=T17."Write", "Y Array In"=w752) -> ("File Info Buffer Out"=w746:T4[], "Y Array Buffer Out"=w748:dbl[][])  [unwired: 8 in, 3 out]
            n341 = for {
              tunnel: w746 -> [w764] mode=indexing
              tunnel: [w763] -> w750 mode=indexing
              n342 = call "X-Axis_Generator_f.vi"("File Info In"=w764) -> ("X-axis  (nm)"=w763:dbl[])  [unwired: 11 in, 7 out]
            }
            n343 = Unbundle By Name(w741) -> ("Exp Index"=w740:u32)
            n344 = Quotient & Remainder(x=w740, y=u32 2) -> (x-y*floor(x/y)=w738:u32)  [unwired: 1 out]
            n345 = Not Equal To 0?(x=w738) -> ()  [unwired: 1 out]
            n346 = case shown="False" "Case Constant\n(See Context Help) 2" {
              tunnel: w737 -> [w760 _]
              frame False {
                n347 = Enqueue Element(queue=w760, element=TRUE) -> ()  [unwired: 2 in, 3 out]
              }
              frame True {
              }
            }
            n348 = Transpose 2D Array(2D array=w750) -> (transposed array=w749:dbl[][])
          }
        }
        n349 = flat-sequence "Cursor delta" {
          frame #0 {
            n350 = property on="Main Data Plot" class="XYGraph (strict)"("Active Cursor"=u32 0, "Active Cursor"=u32 1) -> ("Cursor.Cursor Position:Cursor X"=w727:dbl, "Cursor.Cursor Position:Cursor Y"=w725:dbl, "Cursor.Cursor Position:Cursor X"=w726:dbl, "Cursor.Cursor Position:Cursor Y"=w724:dbl)  [unwired: 2 in, 2 out]
            n351 = Subtract(x=w727, y=w726) -> (x-y=w728:dbl)
            n352 = Subtract(x=w725, y=w724) -> (x-y=w729:dbl)
            n353 = Build Array(w728, w729) -> (→"Cursor delta x & y":dbl[])
          }
        }
        "File Info Buffer Out" <- w694
      }
      event "LoadData?": Value Change {
        n354 = event-data() -> ("NewVal"=w785:bool)  [unwired: 1 in]
        n355 = call "Load Data.vi"("LoadData?"=w785, "File Info Buffer Input"=w786, "Y Array Buffer Input"=w787, "X-Axis Array Input"=w788) -> ("File Info Buffer Out"=w782:T4[], "Data Array output"=w783:dbl[][], "X-Axis Array output"=w784:dbl[][])  [unwired: 1 in, 2 out]
      }
      event "Trace": Value Change {
        n356 = event-data() -> ("NewVal"=w792:bool[])  [unwired: 1 in]
        n357 = Search 1D Array(1D array=w792, element=FALSE) -> (index of element=w790:i32)  [unwired: 1 in]
        n358 = Build Array(w790) -> (w789:i32[])
        n359 = property on="File Info Buffer Out" class="Arr (strict)"("Index Values"=w789) -> ()  [unwired: 2 in, 2 out]
      }
      event "Fixed": Value Change {
        n360 = event-data() -> ()  [unwired: 1 in, 1 out]
        n361 = call "Change Fixed.vi"("Locked Traces"=w806, "Trace Names"=w805) -> ("StoreInto output"=w810:u16, "Pin output"=w802:bool[])  [unwired: 1 in]
        "Pin" <- w802
      }
      event "X-Axis Unit": Value Change {
        n362 = event-data() -> ("NewVal"=w818:u16)  [unwired: 1 in]
        n363 = call-poly "X-Converter_polymorphic.vi"("X-Axis Unit"=w818) -> ("Precision"=w817:i32)  [unwired: 4 in, 3 out]
        n364 = property on="Main Data Plot" class="XYGraph (strict)"("X Scale.Format & Precision:Precision"=w817) -> ()  [unwired: 2 in, 2 out]
      }
      event "Column Headings": Value Change {
        n365 = event-data() -> ("NewVal"=w829:string[])  [unwired: 1 in]
        n366 = for {
          tunnel: w829 -> [w839] mode=indexing
          i -> [w838]
          n367 = property on="Main Data Plot" class="XYGraph (strict)"("Active Plot"=w838, "Plot.Plot Name"=w839) -> ()  [unwired: 2 in, 2 out]
        }
      }
      event "FindAPeaks", "FindBPeaks": Value Change {
        n368 = event-data() -> ()  [unwired: 1 in, 6 out]
        n369 = call-poly "X-Converter_polymorphic.vi"("X-Axis Unit"=w857) -> ("X-Axis Unit String"=w851:string, "Precision"=w852:i32)  [unwired: 4 in, 2 out]
        n370 = Number To Decimal String(number=w852) -> (decimal integer string=w855:string)  [unwired: 1 in]
        n371 = Select(t=u32 0 ("Active Cursor"), s="FindAPeaks", f=u32 1) -> (s? t:f=w846:u32)
        n372 = Concatenate Strings(" ", w851) -> (w849:string)
        n373 = Concatenate Strings("%9.", w855, "f") -> (w850:string)
        n374 = property on="Main Data Plot" class="XYGraph (strict)"("Active Cursor"=w846) -> ("Cursor.Cursor Plot"=w859:i32)  [unwired: 2 in, 2 out]
        n375 = call "PeaksInPlot.vi"("Format String"=w850, "Unit String"=w849, "X-Axis Array"=w863, "Data Array"=w862, "Cursor Plot"=w859) -> ("Peaks: X"=w858:dbl[], "Peak Position Strings []"=w861:string[], "Peaks: Y"=w860:dbl[])
        n376 = case shown="False" "FindBPeaks" {
          tunnel: w861 -> [w873 w875]
          tunnel: w860 -> [w872 w876]
          tunnel: w858 -> [w871 w877]
          tunnel: [w871 w874] -> w843
          tunnel: [w870 w877] -> w842
          tunnel: w841 -> [_ w874]
          tunnel: w840 -> [w870 _]
          frame False {
            n377 = property on="APeakIndex" class="Ring (strict)"("Strings []"=w873) -> ()  [unwired: 2 in, 2 out]
            "A peaks: X" <- w871
            "A peaks: Y" <- w872
          }
          frame True {
            n378 = property on="BPeakIndex" class="Ring (strict)"("Strings []"=w875) -> ()  [unwired: 2 in, 2 out]
            "B peaks: X" <- w877
            "B peaks: Y" <- w876
          }
        }
      }
      event "APeakIndex", "BPeakIndex", "Pressure Unit?": Value Change {
        n379 = event-data() -> ()  [unwired: 1 in, 1 out]
        n380 = call-poly "X-Converter_polymorphic.vi"("X-Axis Unit"=w880) -> ("X-Axis Unit String"=w881:string, "Precision"=w879:i32)  [unwired: 4 in, 2 out]
        n381 = Select(t=2, s="Pressure Unit?", f=w879) -> (s? t:f=w902:i32)
        n382 = Build Array("APeakIndex") -> (w886:u16[])
        n383 = Concatenate Strings(" ", w881) -> (w878:string)
        n384 = Select(t="kb", s="Pressure Unit?", f=w878) -> (s? t:f=w905:string)
        n385 = Build Array("BPeakIndex") -> (w888:u16[])
        n386 = property on="DX" class="DigNum (strict)"("Old Format & Precision:Old Precision"=w902, "Caption.Text"=w905) -> ()  [unwired: 2 in, 2 out]
        n387 = property on="A peaks: Y" class="Arr (strict)"("Index Values"=w886) -> ()  [unwired: 2 in, 2 out]
        n388 = property on="B peaks: X" class="Arr (strict)"("Index Values"=w888) -> ("Index Values"=w893:u32[])  [unwired: 2 in, 2 out]
        n389 = property on="A peaks: X" class="Arr (strict)"("Index Values"=w886) -> ("Index Values"=w889:u32[])  [unwired: 2 in, 2 out]
        n390 = property on="B peaks: Y" class="Arr (strict)"("Index Values"=w888) -> ()  [unwired: 2 in, 2 out]
        n391 = Index Array(array=w889, index=0) -> (element=w891:u32)
        n392 = Index Array(array=w893, index=0) -> (element=w892:u32)
        n393 = Index Array(array=w884, index=w891) -> (element=w895:dbl)
        n394 = Index Array(array=w883, index=w892) -> (element=w896:dbl)
        n395 = Subtract(x=w895, y=w896) -> (x-y=w900:dbl)
        n396 = Select(t=0.0365 ("x-y"), s="Pressure Unit?", f=1.0 ("x-y")) -> (s? t:f=w899:dbl)
        n397 = Divide(x=w900, y=w899) -> (x/y=→"DX":dbl)
      }
      event "Print?": Value Change {
        n398 = event-data() -> ("NewVal"=w915:bool)  [unwired: 1 in]
      }
    }
    n399 = local read "Stop-All"() -> (w660:bool)
    n400 = call "PlotSS.vi"("X-Axis Array (nm) In"=w686, "Mode"=w684, "StoreInto"=w683, "Fixed items"=w677, "X-Axis"=w679, "Data Array In"=w685, "Print"=w680, "File Info Buffer Input"=w687, "Show/hide"=w681, "Data Plot Input"=w670) -> ("X-Axis Array (nm) Out"=w689:dbl[][], "Data Array Out"=w688:dbl[][], "Data Plot"=w672:cluster{dbl[], dbl[]}[], "File Info Buffer Out"=w673:T4[])  [unwired: 2 in]
    "Main Data Plot" <- w672
  }
  n401 = stacked-sequence {
    tunnel: w16 -> [_ _ w927]
    frame #0 {
      n402 = local write "Stop-All"(TRUE ("Stop-All")) -> ()
    }
    frame #1 {
      n403 = Wait (ms)(milliseconds to wait=u32 20000) -> ()  [unwired: 1 out]
    }
    frame #2 {
      n404 = call <vilib>:"Abort Instrument.vi"("VI name"=w927) -> ()  [unwired: 10 in, 1 out]
    }
  }
  n405 = Release Queue(queue=w51, force destroy? (F)=w50) -> ()  [unwired: 1 in, 3 out]
  n406 = Release Queue(queue=w52, force destroy? (F)=w50) -> ()  [unwired: 1 in, 3 out]
